vi "Entrenamiento Fuerza 6.vi"(8 "error in (no error)":errorcluster) -> (0 "error out":errorcluster)   [LabVIEW 2014]
panel:
  out "Tiempo Restante":string="15 : 58"
  out "Tiempo Transcurrido":string="04 : 01"
  in  "Reset":bool
  out "Hola":string="4"
  out "Cluster":T1={"Label"="Start", "Cuadriceps"=0, "Isquiotibiales"=0, "Gluteos"=0, "Abdomen"=0, "Lumbares"=0, "Dorsales"=0, "Trapecio"=0, "Pectorales"=35, "Biceps"=87, "Opcional"=0, "Tiempo"=20, "Impulso"=4, "Ruptura"=1, "Frecuencia"=80, "Profundidad"=200, "Ganancia"=0.1, "Master"=54, "Slider"=0}
  out "Master Ind":string="54%"
  in  "Master":bool
  out "Master?":bool
  out "error out 2":errorcluster={"status"=FALSE, "code"=1073676418, "source"="VISA Close in Entrenamiento Fuerza 6.vi"}
  in  "Puerto Serial":refnum<visa-resource-name>="COM25"
  out "Start?":bool
  in  "Start":bool
  in  "Impulso":bool
  in  "Back":bool
  in  "Help":bool
  in  "Slider":i32(slide) scale=0.0..100.0
  out "Horizontal Graduated Bar":i16(slide) scale=0.0..100.0
  in  "Remove Button":bool
  in  "Add Button":bool
  out "Opcional %":string="0%"
  in  "Opcional Bool":bool
  out "Biceps %":string="87%"
  in  "Biceps Bool":bool
  out "Pectorales %":string="35%"
  in  "Pectorales Bool":bool
  out "Trapecio %":string="0%"
  in  "Trapecio Bool":bool
  out "Dorsales %":string="0%"
  in  "Dorsales Bool":bool
  out "Lumbares %":string="0%"
  in  "Lumbares Bool":bool
  out "Abdomen %":string="0%"
  in  "Abdomen Bool":bool
  out "Gluteos %":string="0%"
  in  "Gluteos Bool":bool
  out "Isquiotibiales %":string="0%"
  in  "Isquiotibiales Bool":bool
  out "Cuadríceps %":string="0%"
  in  "Cuadriceps Bool":bool
  out "date/time string":string="26/11/2015 06:09:03 p. m."
  # "Entrenamiento de Fuerza"
  # "Presentación"
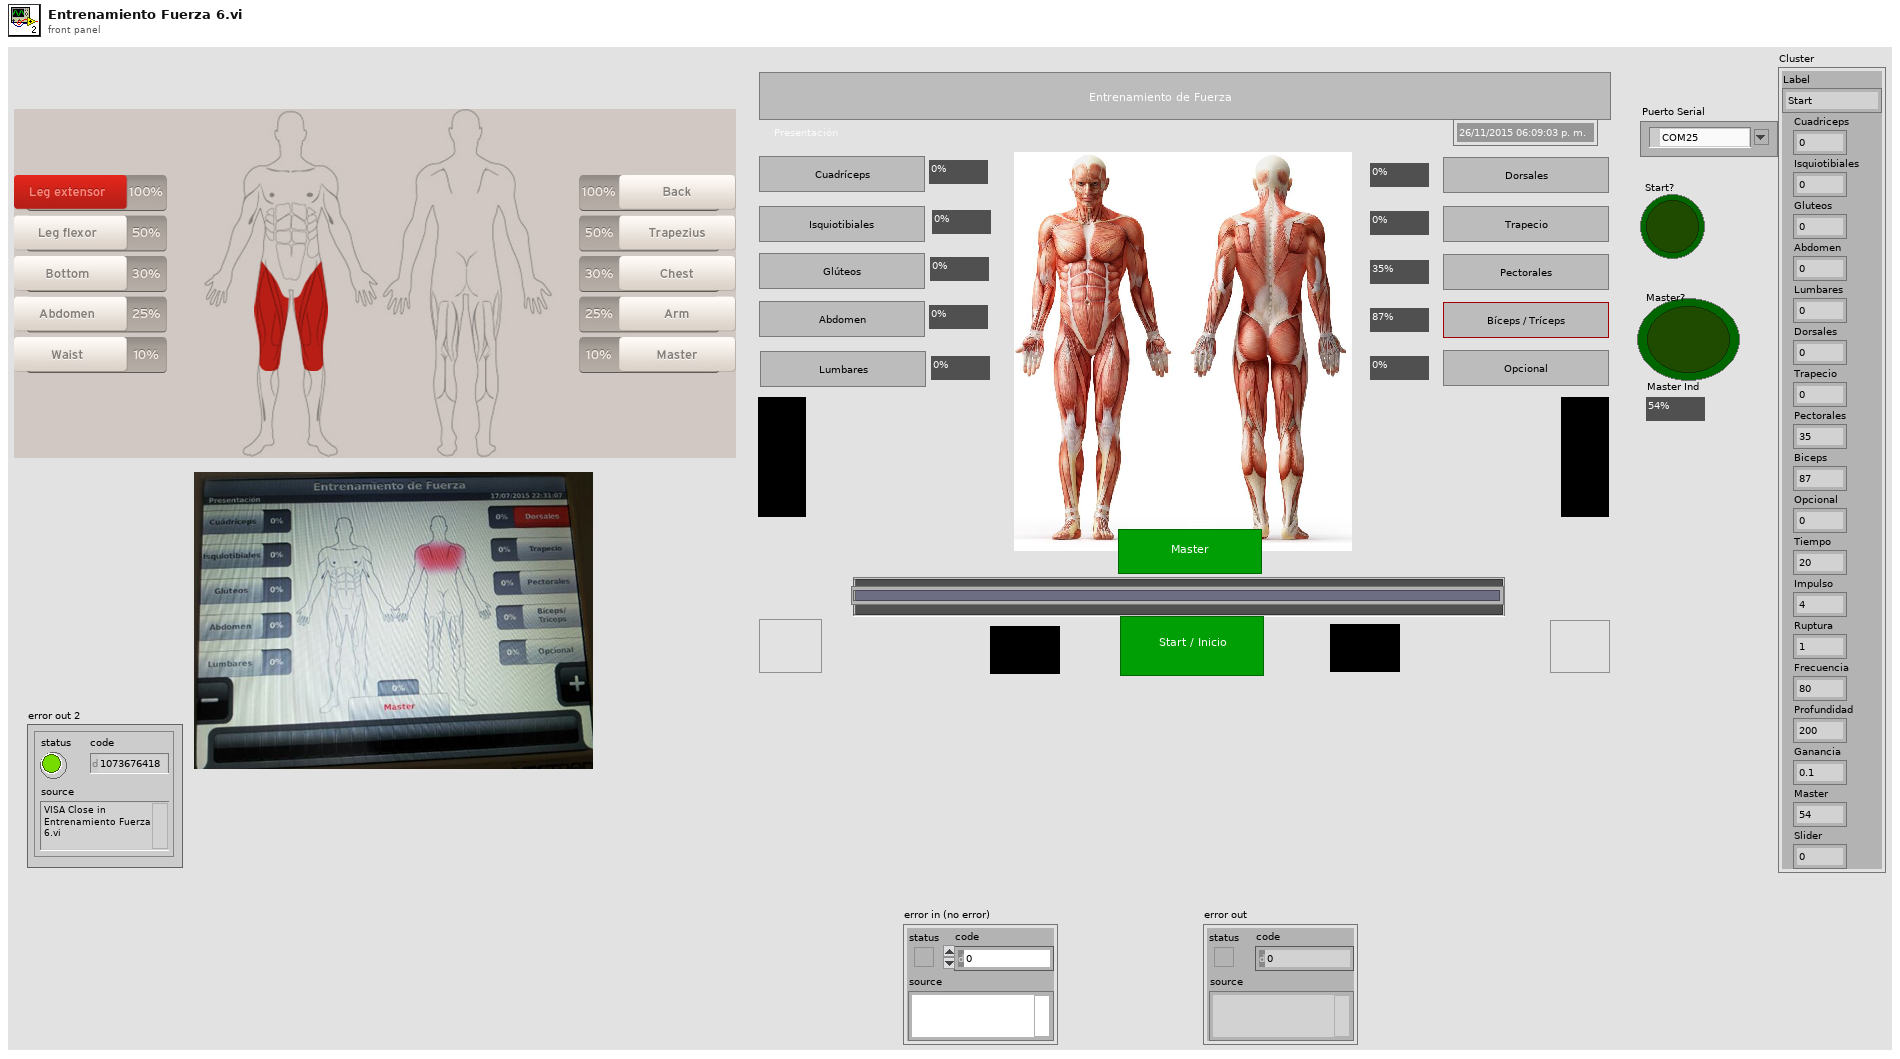
[diagram p1: front panel]
types:
  T1 = cluster{"Label":string, "Cuadriceps":i32, "Isquiotibiales":i32, "Gluteos":i32, "Abdomen":i32, "Lumbares":i32, "Dorsales":i32, "Trapecio":i32, "Pectorales":i32, "Biceps":i32, "Opcional":i32, "Tiempo":i32, "Impulso":i32, "Ruptura":i32, "Frecuencia":i32, "Profundidad":i32, "Ganancia":dbl, "Master":i32, "Slider":i32}
  T2 = cluster{u32, "Boolean Text.Text Colors:Text Color":u32}
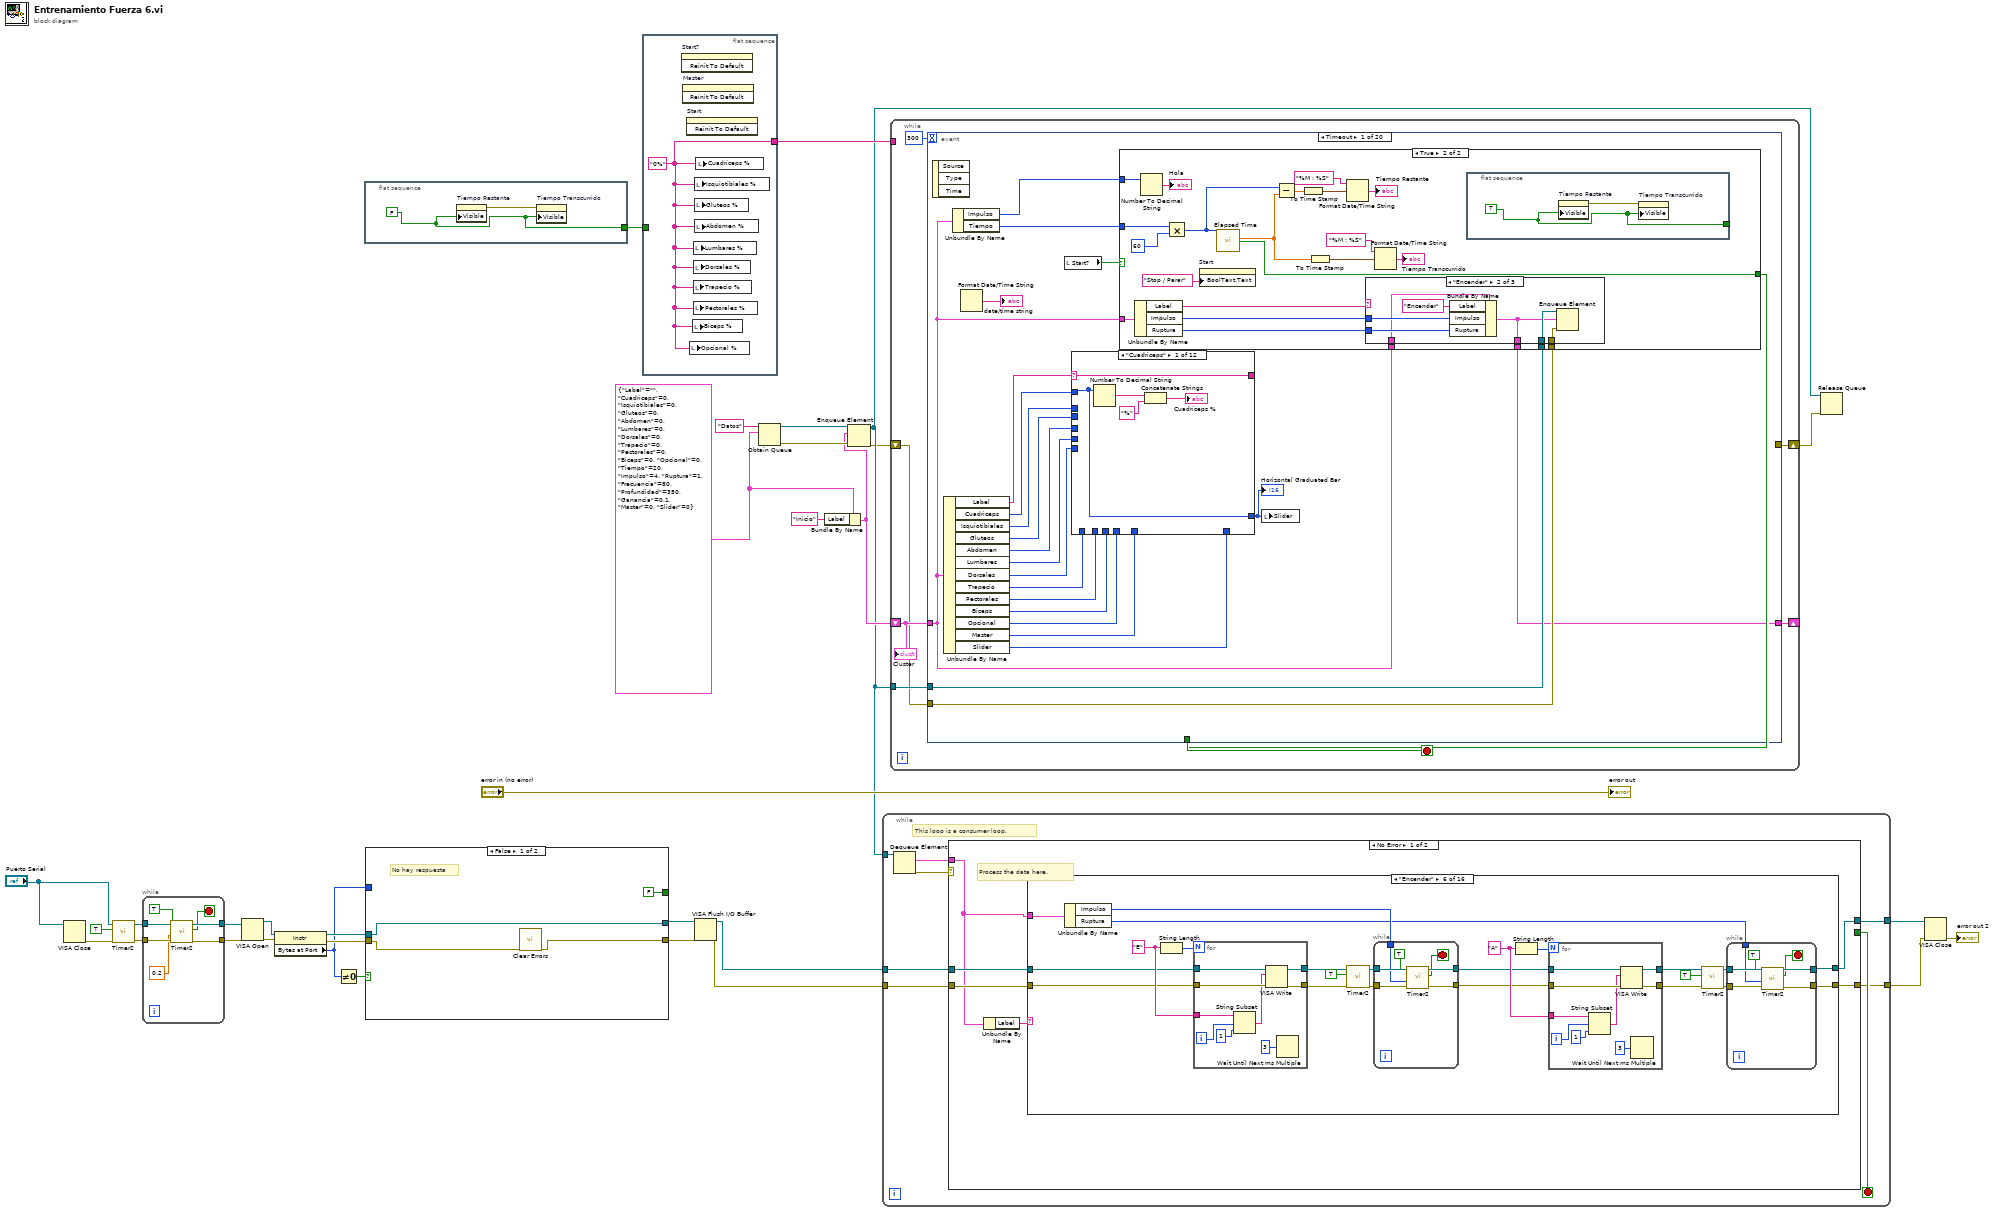
[diagram p0: block diagram]
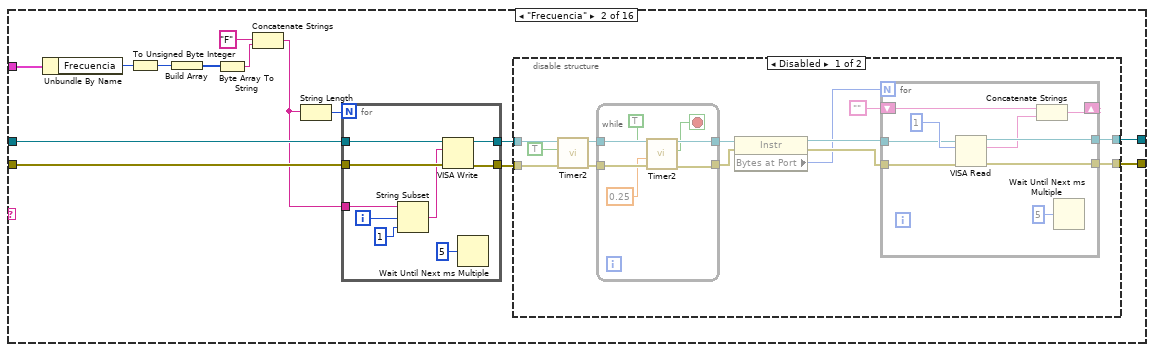
[diagram p3: hidden frame]
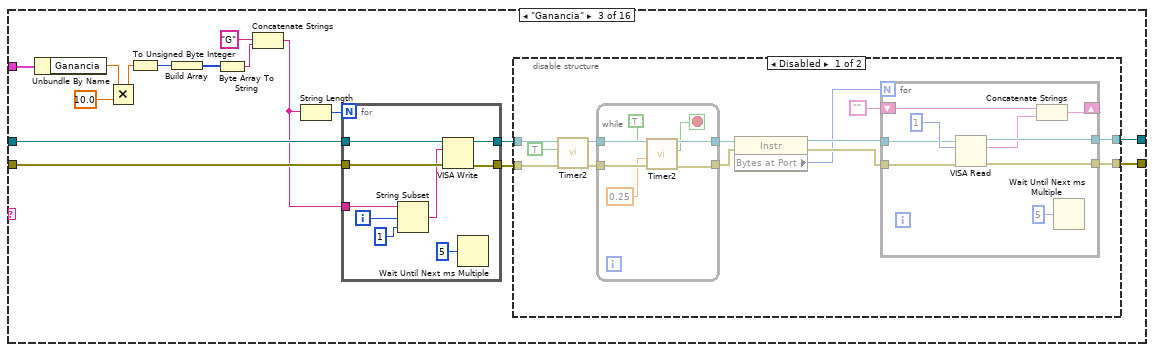
[diagram p5: hidden frame]
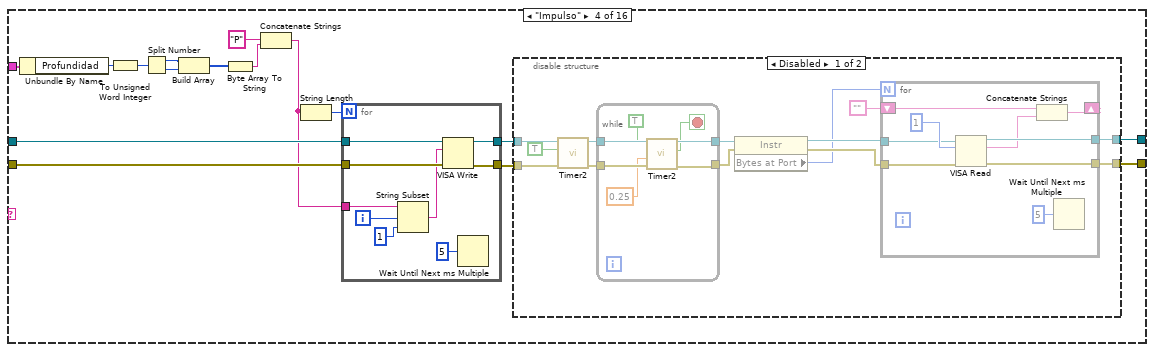
[diagram p7: hidden frame]
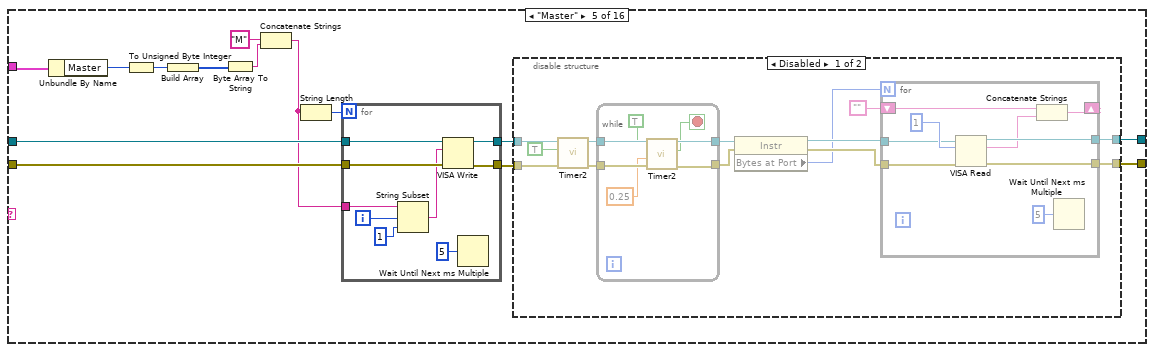
[diagram p9: hidden frame]
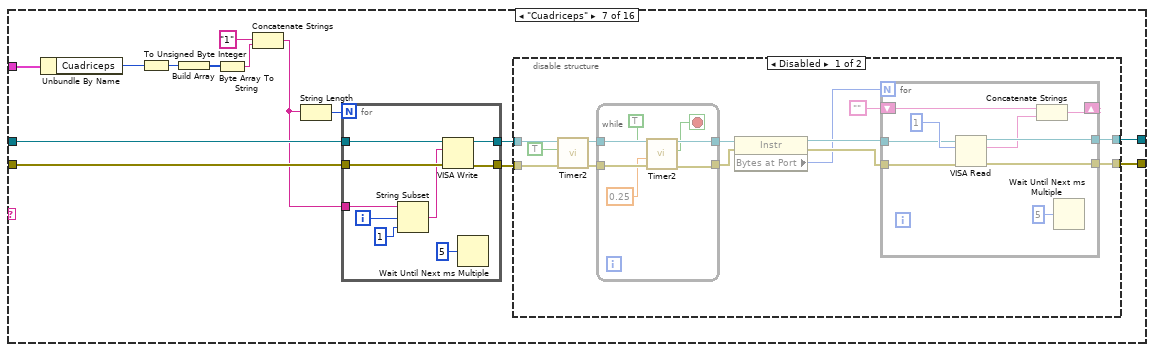
[diagram p11: hidden frame]
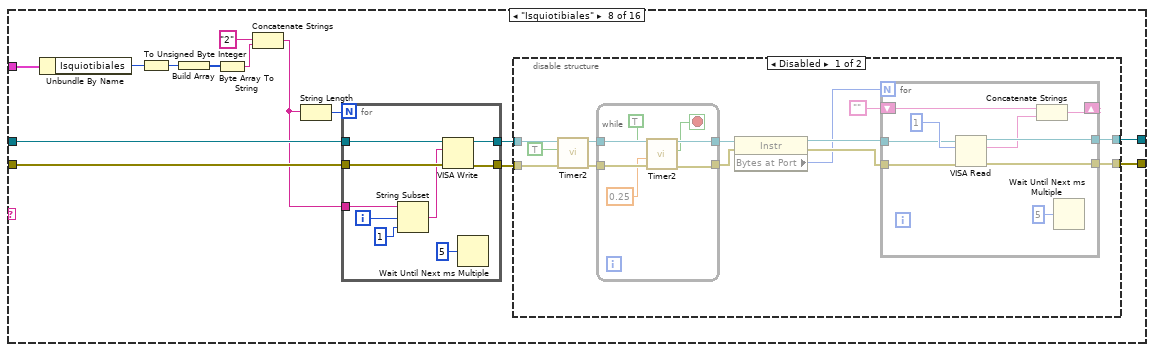
[diagram p13: hidden frame]
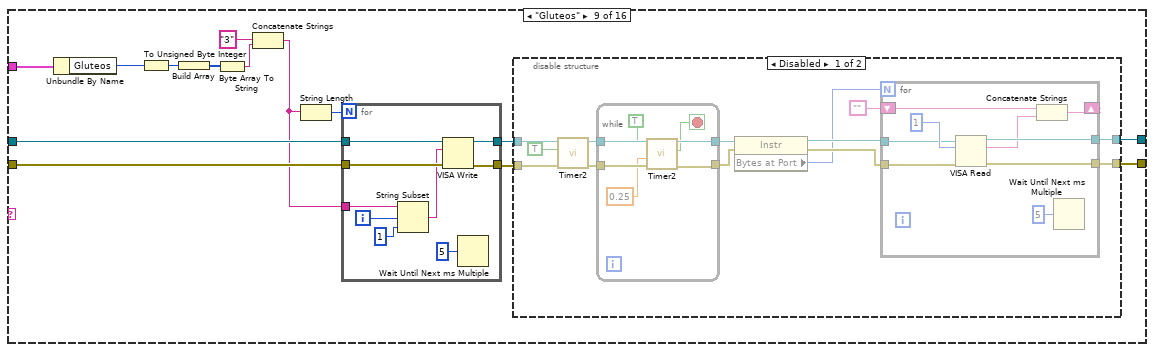
[diagram p15: hidden frame]
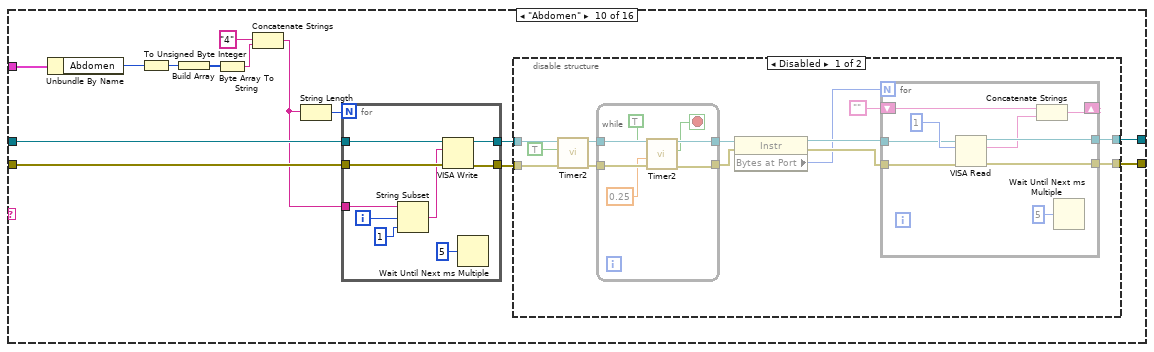
[diagram p17: hidden frame]
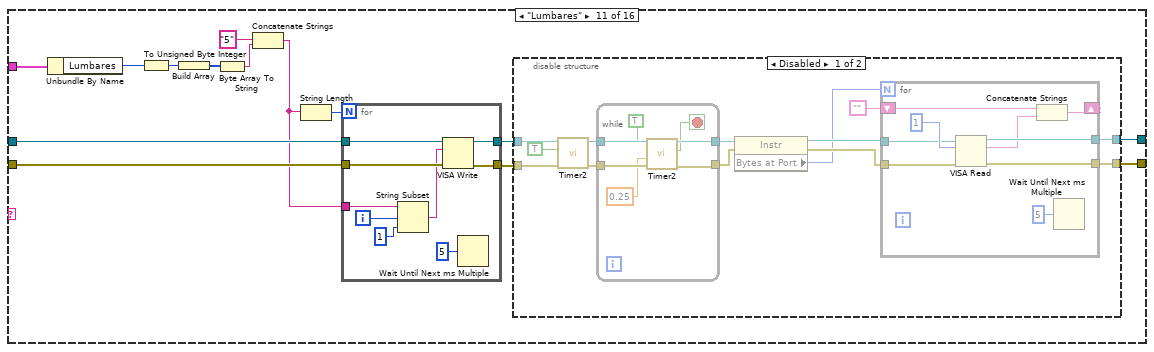
[diagram p19: hidden frame]
diagram:
  w12 = T1 {"Label"="", "Cuadriceps"=0, "Isquiotibiales"=0, "Gluteos"=0, "Abdomen"=0, "Lumbares"=0, "Dorsales"=0, "Trapecio"=0, "Pectorales"=0, "Biceps"=0, "Opcional"=0, "Tiempo"=20, "Impulso"=4, "Ruptura"=1, "Frecuencia"=80, "Profundidad"=350, "Ganancia"=0.1, "Master"=0, "Slider"=0}
  n1 = VISA Close(VISA resource name="Puerto Serial") -> (error out=w27:errorcluster)  [unwired: 1 in]
  n2 = call "Timer2.vi"("error in (no error)"=w27, "Reset"=TRUE) -> ("error out"=w26:errorcluster)  [unwired: 7 in, 2 out]
  n3 = while {
    tunnel: w26 -> [w36]
    tunnel: "Puerto Serial" -> [w37]
    tunnel: [w37] -> w28
    tunnel: [w35] -> w24
    stop <- w34 stop-if-true
    n4 = call "Timer2.vi"("error in (no error)"=w36, "Time Target (s)"=0.2, "Pause"=TRUE) -> ("error out"=w35:errorcluster, "Time has Elapsed"=w34:bool)  [unwired: 6 in, 1 out]
  }
  n5 = VISA Open(error in (no error)=w24, VISA resource name=w28) -> (VISA resource name=w16:refnum<visa-resource-name>, error out=w17:errorcluster)  [unwired: 3 in]
  n6 = property class="Instr"(reference=w16, error in=w17) -> (reference out=w22:refnum<visa-resource-name>, error out=w23:errorcluster, "Bytes at Port"=w20:u32)
  n7 = Not Equal To 0?(x=w20) -> (x != 0?=w21:bool)
  n8 = flat-sequence {
    tunnel: [w38] -> w1
    frame #0 {
      w38 = FALSE ("Visible")
      n9 = property on="Tiempo Restante" class="Str"("Visible"=w38) -> (error out=w39:errorcluster)  [unwired: 2 in, 1 out]
      n10 = property on="Tiempo Transcurrido" class="Str"(error in=w39, "Visible"=w38) -> ()  [unwired: 1 in, 2 out]
    }
  }
  n11 = case shown="False" w21 {
    tunnel: w23 -> [w41 w51]
    tunnel: w22 -> [w43 w50]
    tunnel: w20 -> [_ w49]
    tunnel: [w43 w47] -> w18
    tunnel: [w40 w46] -> w19
    tunnel: [FALSE w45] -> _
    frame False {
      # "No hay respuesta"
      n12 = call <vilib>:"Clear Errors.vi"("error in (no error)"=w41) -> ("error out"=w40:errorcluster)  [unwired: 5 in, 1 out]
    }
    frame True {
      # "Recibe Datos de Respuesta"
      n13 = for {
        N: w49 -> [_]
        tunnel: w51 -> [w60]
        tunnel: w50 -> [w59]
        shift-right: [w54] -> w44
        shift-left: "" -> [w58]
        tunnel: [w57] -> w46
        tunnel: [w56] -> w47
        n14 = VISA Read(VISA resource name=w59, byte count=u32 1, error in (no error)=w60) -> (VISA resource name out=w56:refnum<visa-resource-name>, read buffer=w53:string, error out=w57:errorcluster)  [unwired: 1 out]
        n15 = Concatenate Strings(w58, w53) -> (w54:string)
        n16 = Wait Until Next ms Multiple(millisecond multiple=u32 1) -> ()  [unwired: 1 out]
      }
      n17 = Equal?(x=w44, y="OK") -> (x = y?=w45:bool)
    }
  }
  n18 = flat-sequence {
    tunnel: [w62] -> w15
    tunnel: w1 -> [_]
    frame #0 {
      w62 = "0%" ("Cuadríceps %")
      n19 = invoke on="Start?" class="Bool (strict)" method="Reinit To Default"() -> ()  [unwired: 3 in, 3 out]
      n20 = invoke on="Master" class="Bool (strict)" method="Reinit To Default"() -> ()  [unwired: 3 in, 3 out]
      n21 = invoke on="Start" class="Bool (strict)" method="Reinit To Default"() -> ()  [unwired: 3 in, 3 out]
      n22 = local write "Opcional %"(w62) -> ()
      n23 = local write "Biceps %"(w62) -> ()
      n24 = local write "Trapecio %"(w62) -> ()
      n25 = local write "Pectorales %"(w62) -> ()
      n26 = local write "Lumbares %"(w62) -> ()
      n27 = local write "Dorsales %"(w62) -> ()
      n28 = local write "Isquiotibiales %"(w62) -> ()
      n29 = local write "Gluteos %"(w62) -> ()
      n30 = local write "Abdomen %"(w62) -> ()
      n31 = local write "Cuadríceps %"(w62) -> ()
    }
  }
  n32 = VISA Flush I/O Buffer(VISA resource name=w18, error in (no error)=w19) -> (VISA resource name out=w7:refnum<visa-resource-name>, error out=w6:errorcluster)  [unwired: 1 in]
  n33 = Obtain Queue(name (unnamed)="Datos", element data type=w12) -> (queue out=w13:refnum<queue>, error out=w14:errorcluster)  [unwired: 3 in, 1 out]
  n34 = Bundle By Name(cluster=w12, "Label"="Inicio") -> (w10:T1)
  n35 = Enqueue Element(queue=w13, element=w10, error in (no error)=w14) -> (queue out=w8:refnum<queue>, error out=w3:errorcluster)  [unwired: 1 in, 1 out]
  n36 = while {
    tunnel: w8 -> [w70]
    tunnel: w7 -> [w66]
    tunnel: w6 -> [w65]
    tunnel: [w64] -> w5
    tunnel: [w63] -> w4
    stop <- w67 stop-if-true
    # "This loop is a consumer loop."
    n37 = Dequeue Element(queue=w70) -> (element=w68:T1, error out=w69:errorcluster)  [unwired: 2 in, 2 out]
    n38 = case shown="No Error" w69 {
      tunnel: w68 -> [w71 _]
      tunnel: [_ TRUE] -> w67
      tunnel: w66 -> [w76 w862]
      tunnel: w65 -> [w75 w863]
      tunnel: [w74 w862] -> w64
      tunnel: [w73 w863] -> w63
      frame No Error {
        # "Process the data here."
        n39 = Unbundle By Name(w71) -> ("Label"=w72:string)
        n40 = case shown="\"Encender\"" w72 {
          tunnel: w76 -> [w77 w92 w146 w200 w252 w294 w355 w407 w459 w511 w563 w615 w667 w719 w771 w823]
          tunnel: w75 -> [w78 w91 w145 w199 w251 w293 w354 w406 w458 w510 w562 w614 w666 w718 w770 w822]
          tunnel: [w78 w90 w144 w198 w250 w296 w353 w405 w457 w509 w561 w613 w665 w717 w769 w821] -> w73
          tunnel: [w77 w89 w143 w197 w249 w295 w352 w404 w456 w508 w560 w612 w664 w716 w768 w820] -> w74
          tunnel: w71 -> [_ w81 w136 w190 w239 w311 w344 w396 w448 w500 w552 w604 w656 w708 w760 w812]
          frame "Inicio", Default {
          }
          frame "Frecuencia" {
            n41 = Unbundle By Name(w81) -> ("Frecuencia"=w82:i32)
            n42 = To Unsigned Byte Integer(number=w82) -> (unsigned 8bit integer=w80:u8)
            n43 = Build Array(w80) -> (w79:u8[])
            n44 = Byte Array To String(unsigned byte array=w79) -> (string=w84:string)
            n45 = Concatenate Strings("F", w84) -> (w83:string)
            n46 = String Length(string=w83) -> (length=w88:i32)
            n47 = for {
              N: w88 -> [_]
              tunnel: w91 -> [w130]
              tunnel: w92 -> [w129]
              tunnel: w83 -> [w126]
              tunnel: [w123] -> w86
              tunnel: [w122] -> w87
              i -> [w124]
              n48 = String Subset(string=w126, offset (0)=w124, length (rest)=1 ("length (rest)")) -> (substring=w127:string)
              n49 = VISA Write(VISA resource name=w129, write buffer=w127, error in (no error)=w130) -> (VISA resource name out=w122:refnum<visa-resource-name>, error out=w123:errorcluster)  [unwired: 1 out]
              n50 = Wait Until Next ms Multiple(millisecond multiple=u32 5) -> ()  [unwired: 1 out]
            }
            n51 = disable-structure shown="Disabled" {
              disable-tunnel: [w104 w120] -> w90
              disable-tunnel: [w103 w121] -> w89
              disable-tunnel: w87 -> [w98 w121]
              disable-tunnel: w86 -> [w94 w120]
              frame Disabled {
                n52 = call "Timer2.vi"("error in (no error)"=w94, "Reset"=TRUE) -> ("error out"=w93:errorcluster)  [unwired: 7 in, 2 out]
                n53 = while {
                  tunnel: w98 -> [w110]
                  tunnel: [w110] -> w97
                  tunnel: [w108] -> w96
                  tunnel: w93 -> [w109]
                  stop <- w107 stop-if-true
                  n54 = call "Timer2.vi"("error in (no error)"=w109, "Time Target (s)"=0.25, "Pause"=TRUE) -> ("error out"=w108:errorcluster, "Time has Elapsed"=w107:bool)  [unwired: 6 in, 1 out]
                }
                n55 = property class="Instr"(reference=w97, error in=w96) -> (reference out=w101:refnum<visa-resource-name>, error out=w100:errorcluster, "Bytes at Port"=w99:u32)
                n56 = for {
                  N: w99 -> [_]
                  tunnel: w100 -> [w118]
                  tunnel: w101 -> [w117]
                  shift-right: [w112] -> _
                  shift-left: "" -> [w116]
                  tunnel: [w115] -> w104
                  tunnel: [w114] -> w103
                  n57 = VISA Read(VISA resource name=w117, byte count=u32 1, error in (no error)=w118) -> (VISA resource name out=w114:refnum<visa-resource-name>, read buffer=w111:string, error out=w115:errorcluster)  [unwired: 1 out]
                  n58 = Concatenate Strings(w116, w111) -> (w112:string)
                  n59 = Wait Until Next ms Multiple(millisecond multiple=u32 5) -> ()  [unwired: 1 out]
                }
              }
              frame Enabled {
              }
            }
          }
          frame "Ganancia" {
            n60 = Unbundle By Name(w136) -> ("Ganancia"=w132:dbl)
            n61 = Multiply(x=w132, y=10.0) -> (x*y=w133:dbl)
            n62 = To Unsigned Byte Integer(number=w133) -> (unsigned 8bit integer=w135:u8)
            n63 = Build Array(w135) -> (w134:u8[])
            n64 = Byte Array To String(unsigned byte array=w134) -> (string=w138:string)
            n65 = Concatenate Strings("G", w138) -> (w137:string)
            n66 = String Length(string=w137) -> (length=w142:i32)
            n67 = for {
              N: w142 -> [_]
              tunnel: w145 -> [w184]
              tunnel: w146 -> [w183]
              tunnel: w137 -> [w180]
              tunnel: [w177] -> w140
              tunnel: [w176] -> w141
              i -> [w178]
              n68 = String Subset(string=w180, offset (0)=w178, length (rest)=1 ("length (rest)")) -> (substring=w181:string)
              n69 = VISA Write(VISA resource name=w183, write buffer=w181, error in (no error)=w184) -> (VISA resource name out=w176:refnum<visa-resource-name>, error out=w177:errorcluster)  [unwired: 1 out]
              n70 = Wait Until Next ms Multiple(millisecond multiple=u32 5) -> ()  [unwired: 1 out]
            }
            n71 = disable-structure shown="Disabled" {
              disable-tunnel: [w158 w174] -> w144
              disable-tunnel: [w157 w175] -> w143
              disable-tunnel: w141 -> [w152 w175]
              disable-tunnel: w140 -> [w148 w174]
              frame Disabled {
                n72 = call "Timer2.vi"("error in (no error)"=w148, "Reset"=TRUE) -> ("error out"=w147:errorcluster)  [unwired: 7 in, 2 out]
                n73 = while {
                  tunnel: w152 -> [w164]
                  tunnel: [w164] -> w151
                  tunnel: [w162] -> w150
                  tunnel: w147 -> [w163]
                  stop <- w161 stop-if-true
                  n74 = call "Timer2.vi"("error in (no error)"=w163, "Time Target (s)"=0.25, "Pause"=TRUE) -> ("error out"=w162:errorcluster, "Time has Elapsed"=w161:bool)  [unwired: 6 in, 1 out]
                }
                n75 = property class="Instr"(reference=w151, error in=w150) -> (reference out=w155:refnum<visa-resource-name>, error out=w154:errorcluster, "Bytes at Port"=w153:u32)
                n76 = for {
                  N: w153 -> [_]
                  tunnel: w154 -> [w172]
                  tunnel: w155 -> [w171]
                  shift-right: [w166] -> _
                  shift-left: "" -> [w170]
                  tunnel: [w169] -> w158
                  tunnel: [w168] -> w157
                  n77 = VISA Read(VISA resource name=w171, byte count=u32 1, error in (no error)=w172) -> (VISA resource name out=w168:refnum<visa-resource-name>, read buffer=w165:string, error out=w169:errorcluster)  [unwired: 1 out]
                  n78 = Concatenate Strings(w170, w165) -> (w166:string)
                  n79 = Wait Until Next ms Multiple(millisecond multiple=u32 5) -> ()  [unwired: 1 out]
                }
              }
              frame Enabled {
              }
            }
          }
          frame "Impulso" {
            n80 = Unbundle By Name(w190) -> ("Profundidad"=w187:i32)
            n81 = To Unsigned Word Integer(number=w187) -> (unsigned 16bit integer=w186:u16)
            n82 = Split Number(x=w186) -> (hi(x)=w189:u8, lo(x)=w188:u8)
            n83 = Build Array(w189, w188) -> (w185:u8[])
            n84 = Byte Array To String(unsigned byte array=w185) -> (string=w192:string)
            n85 = Concatenate Strings("P", w192) -> (w191:string)
            n86 = String Length(string=w191) -> (length=w196:i32)
            n87 = for {
              N: w196 -> [_]
              tunnel: w199 -> [w238]
              tunnel: w200 -> [w237]
              tunnel: w191 -> [w234]
              tunnel: [w231] -> w194
              tunnel: [w230] -> w195
              i -> [w232]
              n88 = String Subset(string=w234, offset (0)=w232, length (rest)=1 ("length (rest)")) -> (substring=w235:string)
              n89 = VISA Write(VISA resource name=w237, write buffer=w235, error in (no error)=w238) -> (VISA resource name out=w230:refnum<visa-resource-name>, error out=w231:errorcluster)  [unwired: 1 out]
              n90 = Wait Until Next ms Multiple(millisecond multiple=u32 5) -> ()  [unwired: 1 out]
            }
            n91 = disable-structure shown="Disabled" {
              disable-tunnel: [w212 w228] -> w198
              disable-tunnel: [w211 w229] -> w197
              disable-tunnel: w195 -> [w206 w229]
              disable-tunnel: w194 -> [w202 w228]
              frame Disabled {
                n92 = call "Timer2.vi"("error in (no error)"=w202, "Reset"=TRUE) -> ("error out"=w201:errorcluster)  [unwired: 7 in, 2 out]
                n93 = while {
                  tunnel: w206 -> [w218]
                  tunnel: [w218] -> w205
                  tunnel: [w216] -> w204
                  tunnel: w201 -> [w217]
                  stop <- w215 stop-if-true
                  n94 = call "Timer2.vi"("error in (no error)"=w217, "Time Target (s)"=0.25, "Pause"=TRUE) -> ("error out"=w216:errorcluster, "Time has Elapsed"=w215:bool)  [unwired: 6 in, 1 out]
                }
                n95 = property class="Instr"(reference=w205, error in=w204) -> (reference out=w209:refnum<visa-resource-name>, error out=w208:errorcluster, "Bytes at Port"=w207:u32)
                n96 = for {
                  N: w207 -> [_]
                  tunnel: w208 -> [w226]
                  tunnel: w209 -> [w225]
                  shift-right: [w220] -> _
                  shift-left: "" -> [w224]
                  tunnel: [w223] -> w212
                  tunnel: [w222] -> w211
                  n97 = VISA Read(VISA resource name=w225, byte count=u32 1, error in (no error)=w226) -> (VISA resource name out=w222:refnum<visa-resource-name>, read buffer=w219:string, error out=w223:errorcluster)  [unwired: 1 out]
                  n98 = Concatenate Strings(w224, w219) -> (w220:string)
                  n99 = Wait Until Next ms Multiple(millisecond multiple=u32 5) -> ()  [unwired: 1 out]
                }
              }
              frame Enabled {
              }
            }
          }
          frame "Master" {
            n100 = Unbundle By Name(w239) -> ("Master"=w242:i32)
            n101 = To Unsigned Byte Integer(number=w242) -> (unsigned 8bit integer=w241:u8)
            n102 = Build Array(w241) -> (w240:u8[])
            n103 = Byte Array To String(unsigned byte array=w240) -> (string=w244:string)
            n104 = Concatenate Strings("M", w244) -> (w243:string)
            n105 = String Length(string=w243) -> (length=w248:i32)
            n106 = for {
              N: w248 -> [_]
              tunnel: w251 -> [w290]
              tunnel: w252 -> [w289]
              tunnel: w243 -> [w286]
              tunnel: [w283] -> w246
              tunnel: [w282] -> w247
              i -> [w284]
              n107 = String Subset(string=w286, offset (0)=w284, length (rest)=1 ("length (rest)")) -> (substring=w287:string)
              n108 = VISA Write(VISA resource name=w289, write buffer=w287, error in (no error)=w290) -> (VISA resource name out=w282:refnum<visa-resource-name>, error out=w283:errorcluster)  [unwired: 1 out]
              n109 = Wait Until Next ms Multiple(millisecond multiple=u32 5) -> ()  [unwired: 1 out]
            }
            n110 = disable-structure shown="Disabled" {
              disable-tunnel: [w264 w280] -> w250
              disable-tunnel: [w263 w281] -> w249
              disable-tunnel: w247 -> [w258 w281]
              disable-tunnel: w246 -> [w254 w280]
              frame Disabled {
                n111 = call "Timer2.vi"("error in (no error)"=w254, "Reset"=TRUE) -> ("error out"=w253:errorcluster)  [unwired: 7 in, 2 out]
                n112 = while {
                  tunnel: w258 -> [w270]
                  tunnel: [w270] -> w257
                  tunnel: [w268] -> w256
                  tunnel: w253 -> [w269]
                  stop <- w267 stop-if-true
                  n113 = call "Timer2.vi"("error in (no error)"=w269, "Time Target (s)"=0.25, "Pause"=TRUE) -> ("error out"=w268:errorcluster, "Time has Elapsed"=w267:bool)  [unwired: 6 in, 1 out]
                }
                n114 = property class="Instr"(reference=w257, error in=w256) -> (reference out=w261:refnum<visa-resource-name>, error out=w260:errorcluster, "Bytes at Port"=w259:u32)
                n115 = for {
                  N: w259 -> [_]
                  tunnel: w260 -> [w278]
                  tunnel: w261 -> [w277]
                  shift-right: [w272] -> _
                  shift-left: "" -> [w276]
                  tunnel: [w275] -> w264
                  tunnel: [w274] -> w263
                  n116 = VISA Read(VISA resource name=w277, byte count=u32 1, error in (no error)=w278) -> (VISA resource name out=w274:refnum<visa-resource-name>, read buffer=w271:string, error out=w275:errorcluster)  [unwired: 1 out]
                  n117 = Concatenate Strings(w276, w271) -> (w272:string)
                  n118 = Wait Until Next ms Multiple(millisecond multiple=u32 5) -> ()  [unwired: 1 out]
                }
              }
              frame Enabled {
              }
            }
          }
          frame "Encender" {
            w301 = "A"
            w307 = "E"
            n119 = Unbundle By Name(w311) -> ("Impulso"=w292:i32, "Ruptura"=w291:i32)
            n120 = String Length(string=w307) -> (length=w310:i32)
            n121 = for {
              N: w310 -> [_]
              tunnel: w293 -> [w341]
              tunnel: w294 -> [w340]
              tunnel: w307 -> [w337]
              tunnel: [w334] -> w308
              tunnel: [w333] -> w309
              i -> [w335]
              n122 = String Subset(string=w337, offset (0)=w335, length (rest)=1 ("length (rest)")) -> (substring=w338:string)
              n123 = VISA Write(VISA resource name=w340, write buffer=w338, error in (no error)=w341) -> (VISA resource name out=w333:refnum<visa-resource-name>, error out=w334:errorcluster)  [unwired: 1 out]
              n124 = Wait Until Next ms Multiple(millisecond multiple=u32 3) -> ()  [unwired: 1 out]
            }
            n125 = call "Timer2.vi"("error in (no error)"=w308, "Reset"=TRUE) -> ("error out"=w305:errorcluster)  [unwired: 7 in, 2 out]
            n126 = while {
              tunnel: w309 -> [w332]
              tunnel: [w332] -> w298
              tunnel: [w330] -> w297
              tunnel: w305 -> [w331]
              tunnel: w292 -> [w327]
              stop <- w329 stop-if-true
              n127 = call "Timer2.vi"("error in (no error)"=w331, "Time Target (s)"=w327, "Pause"=TRUE) -> ("error out"=w330:errorcluster, "Time has Elapsed"=w329:bool)  [unwired: 6 in, 1 out]
            }
            n128 = String Length(string=w301) -> (length=w304:i32)
            n129 = for {
              N: w304 -> [_]
              tunnel: w297 -> [w326]
              tunnel: w298 -> [w325]
              tunnel: w301 -> [w322]
              tunnel: [w319] -> w302
              tunnel: [w318] -> w303
              i -> [w320]
              n130 = String Subset(string=w322, offset (0)=w320, length (rest)=1 ("length (rest)")) -> (substring=w323:string)
              n131 = VISA Write(VISA resource name=w325, write buffer=w323, error in (no error)=w326) -> (VISA resource name out=w318:refnum<visa-resource-name>, error out=w319:errorcluster)  [unwired: 1 out]
              n132 = Wait Until Next ms Multiple(millisecond multiple=u32 3) -> ()  [unwired: 1 out]
            }
            n133 = call "Timer2.vi"("error in (no error)"=w302, "Reset"=TRUE) -> ("error out"=w299:errorcluster)  [unwired: 7 in, 2 out]
            n134 = while {
              tunnel: w303 -> [w317]
              tunnel: [w317] -> w295
              tunnel: [w315] -> w296
              tunnel: w299 -> [w316]
              tunnel: w291 -> [w312]
              stop <- w314 stop-if-true
              n135 = call "Timer2.vi"("error in (no error)"=w316, "Time Target (s)"=w312, "Pause"=TRUE) -> ("error out"=w315:errorcluster, "Time has Elapsed"=w314:bool)  [unwired: 6 in, 1 out]
            }
          }
          frame "Cuadriceps" {
            n136 = Unbundle By Name(w344) -> ("Cuadriceps"=w342:i32)
            n137 = To Unsigned Byte Integer(number=w342) -> (unsigned 8bit integer=w343:u8)
            n138 = Build Array(w343) -> (w348:u8[])
            n139 = Byte Array To String(unsigned byte array=w348) -> (string=w346:string)
            n140 = Concatenate Strings("1", w346) -> (w345:string)
            n141 = String Length(string=w345) -> (length=w351:i32)
            n142 = for {
              N: w351 -> [_]
              tunnel: w354 -> [w393]
              tunnel: w355 -> [w392]
              tunnel: w345 -> [w389]
              tunnel: [w386] -> w349
              tunnel: [w385] -> w350
              i -> [w387]
              n143 = String Subset(string=w389, offset (0)=w387, length (rest)=1 ("length (rest)")) -> (substring=w390:string)
              n144 = VISA Write(VISA resource name=w392, write buffer=w390, error in (no error)=w393) -> (VISA resource name out=w385:refnum<visa-resource-name>, error out=w386:errorcluster)  [unwired: 1 out]
              n145 = Wait Until Next ms Multiple(millisecond multiple=u32 5) -> ()  [unwired: 1 out]
            }
            n146 = disable-structure shown="Disabled" {
              disable-tunnel: [w367 w383] -> w353
              disable-tunnel: [w366 w384] -> w352
              disable-tunnel: w350 -> [w361 w384]
              disable-tunnel: w349 -> [w357 w383]
              frame Disabled {
                n147 = call "Timer2.vi"("error in (no error)"=w357, "Reset"=TRUE) -> ("error out"=w356:errorcluster)  [unwired: 7 in, 2 out]
                n148 = while {
                  tunnel: w361 -> [w373]
                  tunnel: [w373] -> w360
                  tunnel: [w371] -> w359
                  tunnel: w356 -> [w372]
                  stop <- w370 stop-if-true
                  n149 = call "Timer2.vi"("error in (no error)"=w372, "Time Target (s)"=0.25, "Pause"=TRUE) -> ("error out"=w371:errorcluster, "Time has Elapsed"=w370:bool)  [unwired: 6 in, 1 out]
                }
                n150 = property class="Instr"(reference=w360, error in=w359) -> (reference out=w364:refnum<visa-resource-name>, error out=w363:errorcluster, "Bytes at Port"=w362:u32)
                n151 = for {
                  N: w362 -> [_]
                  tunnel: w363 -> [w381]
                  tunnel: w364 -> [w380]
                  shift-right: [w375] -> _
                  shift-left: "" -> [w379]
                  tunnel: [w378] -> w367
                  tunnel: [w377] -> w366
                  n152 = VISA Read(VISA resource name=w380, byte count=u32 1, error in (no error)=w381) -> (VISA resource name out=w377:refnum<visa-resource-name>, read buffer=w374:string, error out=w378:errorcluster)  [unwired: 1 out]
                  n153 = Concatenate Strings(w379, w374) -> (w375:string)
                  n154 = Wait Until Next ms Multiple(millisecond multiple=u32 5) -> ()  [unwired: 1 out]
                }
              }
              frame Enabled {
              }
            }
          }
          frame "Isquiotibiales" {
            n155 = Unbundle By Name(w396) -> ("Isquiotibiales"=w394:i32)
            n156 = To Unsigned Byte Integer(number=w394) -> (unsigned 8bit integer=w395:u8)
            n157 = Build Array(w395) -> (w400:u8[])
            n158 = Byte Array To String(unsigned byte array=w400) -> (string=w398:string)
            n159 = Concatenate Strings("2", w398) -> (w397:string)
            n160 = String Length(string=w397) -> (length=w403:i32)
            n161 = for {
              N: w403 -> [_]
              tunnel: w406 -> [w445]
              tunnel: w407 -> [w444]
              tunnel: w397 -> [w441]
              tunnel: [w438] -> w401
              tunnel: [w437] -> w402
              i -> [w439]
              n162 = String Subset(string=w441, offset (0)=w439, length (rest)=1 ("length (rest)")) -> (substring=w442:string)
              n163 = VISA Write(VISA resource name=w444, write buffer=w442, error in (no error)=w445) -> (VISA resource name out=w437:refnum<visa-resource-name>, error out=w438:errorcluster)  [unwired: 1 out]
              n164 = Wait Until Next ms Multiple(millisecond multiple=u32 5) -> ()  [unwired: 1 out]
            }
            n165 = disable-structure shown="Disabled" {
              disable-tunnel: [w419 w435] -> w405
              disable-tunnel: [w418 w436] -> w404
              disable-tunnel: w402 -> [w413 w436]
              disable-tunnel: w401 -> [w409 w435]
              frame Disabled {
                n166 = call "Timer2.vi"("error in (no error)"=w409, "Reset"=TRUE) -> ("error out"=w408:errorcluster)  [unwired: 7 in, 2 out]
                n167 = while {
                  tunnel: w413 -> [w425]
                  tunnel: [w425] -> w412
                  tunnel: [w423] -> w411
                  tunnel: w408 -> [w424]
                  stop <- w422 stop-if-true
                  n168 = call "Timer2.vi"("error in (no error)"=w424, "Time Target (s)"=0.25, "Pause"=TRUE) -> ("error out"=w423:errorcluster, "Time has Elapsed"=w422:bool)  [unwired: 6 in, 1 out]
                }
                n169 = property class="Instr"(reference=w412, error in=w411) -> (reference out=w416:refnum<visa-resource-name>, error out=w415:errorcluster, "Bytes at Port"=w414:u32)
                n170 = for {
                  N: w414 -> [_]
                  tunnel: w415 -> [w433]
                  tunnel: w416 -> [w432]
                  shift-right: [w427] -> _
                  shift-left: "" -> [w431]
                  tunnel: [w430] -> w419
                  tunnel: [w429] -> w418
                  n171 = VISA Read(VISA resource name=w432, byte count=u32 1, error in (no error)=w433) -> (VISA resource name out=w429:refnum<visa-resource-name>, read buffer=w426:string, error out=w430:errorcluster)  [unwired: 1 out]
                  n172 = Concatenate Strings(w431, w426) -> (w427:string)
                  n173 = Wait Until Next ms Multiple(millisecond multiple=u32 5) -> ()  [unwired: 1 out]
                }
              }
              frame Enabled {
              }
            }
          }
          frame "Gluteos" {
            n174 = Unbundle By Name(w448) -> ("Gluteos"=w446:i32)
            n175 = To Unsigned Byte Integer(number=w446) -> (unsigned 8bit integer=w447:u8)
            n176 = Build Array(w447) -> (w452:u8[])
            n177 = Byte Array To String(unsigned byte array=w452) -> (string=w450:string)
            n178 = Concatenate Strings("3", w450) -> (w449:string)
            n179 = String Length(string=w449) -> (length=w455:i32)
            n180 = for {
              N: w455 -> [_]
              tunnel: w458 -> [w497]
              tunnel: w459 -> [w496]
              tunnel: w449 -> [w493]
              tunnel: [w490] -> w453
              tunnel: [w489] -> w454
              i -> [w491]
              n181 = String Subset(string=w493, offset (0)=w491, length (rest)=1 ("length (rest)")) -> (substring=w494:string)
              n182 = VISA Write(VISA resource name=w496, write buffer=w494, error in (no error)=w497) -> (VISA resource name out=w489:refnum<visa-resource-name>, error out=w490:errorcluster)  [unwired: 1 out]
              n183 = Wait Until Next ms Multiple(millisecond multiple=u32 5) -> ()  [unwired: 1 out]
            }
            n184 = disable-structure shown="Disabled" {
              disable-tunnel: [w471 w487] -> w457
              disable-tunnel: [w470 w488] -> w456
              disable-tunnel: w454 -> [w465 w488]
              disable-tunnel: w453 -> [w461 w487]
              frame Disabled {
                n185 = call "Timer2.vi"("error in (no error)"=w461, "Reset"=TRUE) -> ("error out"=w460:errorcluster)  [unwired: 7 in, 2 out]
                n186 = while {
                  tunnel: w465 -> [w477]
                  tunnel: [w477] -> w464
                  tunnel: [w475] -> w463
                  tunnel: w460 -> [w476]
                  stop <- w474 stop-if-true
                  n187 = call "Timer2.vi"("error in (no error)"=w476, "Time Target (s)"=0.25, "Pause"=TRUE) -> ("error out"=w475:errorcluster, "Time has Elapsed"=w474:bool)  [unwired: 6 in, 1 out]
                }
                n188 = property class="Instr"(reference=w464, error in=w463) -> (reference out=w468:refnum<visa-resource-name>, error out=w467:errorcluster, "Bytes at Port"=w466:u32)
                n189 = for {
                  N: w466 -> [_]
                  tunnel: w467 -> [w485]
                  tunnel: w468 -> [w484]
                  shift-right: [w479] -> _
                  shift-left: "" -> [w483]
                  tunnel: [w482] -> w471
                  tunnel: [w481] -> w470
                  n190 = VISA Read(VISA resource name=w484, byte count=u32 1, error in (no error)=w485) -> (VISA resource name out=w481:refnum<visa-resource-name>, read buffer=w478:string, error out=w482:errorcluster)  [unwired: 1 out]
                  n191 = Concatenate Strings(w483, w478) -> (w479:string)
                  n192 = Wait Until Next ms Multiple(millisecond multiple=u32 5) -> ()  [unwired: 1 out]
                }
              }
              frame Enabled {
              }
            }
          }
          frame "Abdomen" {
            n193 = Unbundle By Name(w500) -> ("Abdomen"=w498:i32)
            n194 = To Unsigned Byte Integer(number=w498) -> (unsigned 8bit integer=w499:u8)
            n195 = Build Array(w499) -> (w504:u8[])
            n196 = Byte Array To String(unsigned byte array=w504) -> (string=w502:string)
            n197 = Concatenate Strings("4", w502) -> (w501:string)
            n198 = String Length(string=w501) -> (length=w507:i32)
            n199 = for {
              N: w507 -> [_]
              tunnel: w510 -> [w549]
              tunnel: w511 -> [w548]
              tunnel: w501 -> [w545]
              tunnel: [w542] -> w505
              tunnel: [w541] -> w506
              i -> [w543]
              n200 = String Subset(string=w545, offset (0)=w543, length (rest)=1 ("length (rest)")) -> (substring=w546:string)
              n201 = VISA Write(VISA resource name=w548, write buffer=w546, error in (no error)=w549) -> (VISA resource name out=w541:refnum<visa-resource-name>, error out=w542:errorcluster)  [unwired: 1 out]
              n202 = Wait Until Next ms Multiple(millisecond multiple=u32 5) -> ()  [unwired: 1 out]
            }
            n203 = disable-structure shown="Disabled" {
              disable-tunnel: [w523 w539] -> w509
              disable-tunnel: [w522 w540] -> w508
              disable-tunnel: w506 -> [w517 w540]
              disable-tunnel: w505 -> [w513 w539]
              frame Disabled {
                n204 = call "Timer2.vi"("error in (no error)"=w513, "Reset"=TRUE) -> ("error out"=w512:errorcluster)  [unwired: 7 in, 2 out]
                n205 = while {
                  tunnel: w517 -> [w529]
                  tunnel: [w529] -> w516
                  tunnel: [w527] -> w515
                  tunnel: w512 -> [w528]
                  stop <- w526 stop-if-true
                  n206 = call "Timer2.vi"("error in (no error)"=w528, "Time Target (s)"=0.25, "Pause"=TRUE) -> ("error out"=w527:errorcluster, "Time has Elapsed"=w526:bool)  [unwired: 6 in, 1 out]
                }
                n207 = property class="Instr"(reference=w516, error in=w515) -> (reference out=w520:refnum<visa-resource-name>, error out=w519:errorcluster, "Bytes at Port"=w518:u32)
                n208 = for {
                  N: w518 -> [_]
                  tunnel: w519 -> [w537]
                  tunnel: w520 -> [w536]
                  shift-right: [w531] -> _
                  shift-left: "" -> [w535]
                  tunnel: [w534] -> w523
                  tunnel: [w533] -> w522
                  n209 = VISA Read(VISA resource name=w536, byte count=u32 1, error in (no error)=w537) -> (VISA resource name out=w533:refnum<visa-resource-name>, read buffer=w530:string, error out=w534:errorcluster)  [unwired: 1 out]
                  n210 = Concatenate Strings(w535, w530) -> (w531:string)
                  n211 = Wait Until Next ms Multiple(millisecond multiple=u32 5) -> ()  [unwired: 1 out]
                }
              }
              frame Enabled {
              }
            }
          }
          frame "Lumbares" {
            n212 = Unbundle By Name(w552) -> ("Lumbares"=w550:i32)
            n213 = To Unsigned Byte Integer(number=w550) -> (unsigned 8bit integer=w551:u8)
            n214 = Build Array(w551) -> (w556:u8[])
            n215 = Byte Array To String(unsigned byte array=w556) -> (string=w554:string)
            n216 = Concatenate Strings("5", w554) -> (w553:string)
            n217 = String Length(string=w553) -> (length=w559:i32)
            n218 = for {
              N: w559 -> [_]
              tunnel: w562 -> [w601]
              tunnel: w563 -> [w600]
              tunnel: w553 -> [w597]
              tunnel: [w594] -> w557
              tunnel: [w593] -> w558
              i -> [w595]
              n219 = String Subset(string=w597, offset (0)=w595, length (rest)=1 ("length (rest)")) -> (substring=w598:string)
              n220 = VISA Write(VISA resource name=w600, write buffer=w598, error in (no error)=w601) -> (VISA resource name out=w593:refnum<visa-resource-name>, error out=w594:errorcluster)  [unwired: 1 out]
              n221 = Wait Until Next ms Multiple(millisecond multiple=u32 5) -> ()  [unwired: 1 out]
            }
            n222 = disable-structure shown="Disabled" {
              disable-tunnel: [w575 w591] -> w561
              disable-tunnel: [w574 w592] -> w560
              disable-tunnel: w558 -> [w569 w592]
              disable-tunnel: w557 -> [w565 w591]
              frame Disabled {
                n223 = call "Timer2.vi"("error in (no error)"=w565, "Reset"=TRUE) -> ("error out"=w564:errorcluster)  [unwired: 7 in, 2 out]
                n224 = while {
                  tunnel: w569 -> [w581]
                  tunnel: [w581] -> w568
                  tunnel: [w579] -> w567
                  tunnel: w564 -> [w580]
                  stop <- w578 stop-if-true
                  n225 = call "Timer2.vi"("error in (no error)"=w580, "Time Target (s)"=0.25, "Pause"=TRUE) -> ("error out"=w579:errorcluster, "Time has Elapsed"=w578:bool)  [unwired: 6 in, 1 out]
                }
                n226 = property class="Instr"(reference=w568, error in=w567) -> (reference out=w572:refnum<visa-resource-name>, error out=w571:errorcluster, "Bytes at Port"=w570:u32)
                n227 = for {
                  N: w570 -> [_]
                  tunnel: w571 -> [w589]
                  tunnel: w572 -> [w588]
                  shift-right: [w583] -> _
                  shift-left: "" -> [w587]
                  tunnel: [w586] -> w575
                  tunnel: [w585] -> w574
                  n228 = VISA Read(VISA resource name=w588, byte count=u32 1, error in (no error)=w589) -> (VISA resource name out=w585:refnum<visa-resource-name>, read buffer=w582:string, error out=w586:errorcluster)  [unwired: 1 out]
                  n229 = Concatenate Strings(w587, w582) -> (w583:string)
                  n230 = Wait Until Next ms Multiple(millisecond multiple=u32 5) -> ()  [unwired: 1 out]
                }
              }
              frame Enabled {
              }
            }
          }
          frame "Dorsales" {
            n231 = Unbundle By Name(w604) -> ("Dorsales"=w602:i32)
            n232 = To Unsigned Byte Integer(number=w602) -> (unsigned 8bit integer=w603:u8)
            n233 = Build Array(w603) -> (w608:u8[])
            n234 = Byte Array To String(unsigned byte array=w608) -> (string=w606:string)
            n235 = Concatenate Strings("6", w606) -> (w605:string)
            n236 = String Length(string=w605) -> (length=w611:i32)
            n237 = for {
              N: w611 -> [_]
              tunnel: w614 -> [w653]
              tunnel: w615 -> [w652]
              tunnel: w605 -> [w649]
              tunnel: [w646] -> w609
              tunnel: [w645] -> w610
              i -> [w647]
              n238 = String Subset(string=w649, offset (0)=w647, length (rest)=1 ("length (rest)")) -> (substring=w650:string)
              n239 = VISA Write(VISA resource name=w652, write buffer=w650, error in (no error)=w653) -> (VISA resource name out=w645:refnum<visa-resource-name>, error out=w646:errorcluster)  [unwired: 1 out]
              n240 = Wait Until Next ms Multiple(millisecond multiple=u32 5) -> ()  [unwired: 1 out]
            }
            n241 = disable-structure shown="Disabled" {
              disable-tunnel: [w627 w643] -> w613
              disable-tunnel: [w626 w644] -> w612
              disable-tunnel: w610 -> [w621 w644]
              disable-tunnel: w609 -> [w617 w643]
              frame Disabled {
                n242 = call "Timer2.vi"("error in (no error)"=w617, "Reset"=TRUE) -> ("error out"=w616:errorcluster)  [unwired: 7 in, 2 out]
                n243 = while {
                  tunnel: w621 -> [w633]
                  tunnel: [w633] -> w620
                  tunnel: [w631] -> w619
                  tunnel: w616 -> [w632]
                  stop <- w630 stop-if-true
                  n244 = call "Timer2.vi"("error in (no error)"=w632, "Time Target (s)"=0.25, "Pause"=TRUE) -> ("error out"=w631:errorcluster, "Time has Elapsed"=w630:bool)  [unwired: 6 in, 1 out]
                }
                n245 = property class="Instr"(reference=w620, error in=w619) -> (reference out=w624:refnum<visa-resource-name>, error out=w623:errorcluster, "Bytes at Port"=w622:u32)
                n246 = for {
                  N: w622 -> [_]
                  tunnel: w623 -> [w641]
                  tunnel: w624 -> [w640]
                  shift-right: [w635] -> _
                  shift-left: "" -> [w639]
                  tunnel: [w638] -> w627
                  tunnel: [w637] -> w626
                  n247 = VISA Read(VISA resource name=w640, byte count=u32 1, error in (no error)=w641) -> (VISA resource name out=w637:refnum<visa-resource-name>, read buffer=w634:string, error out=w638:errorcluster)  [unwired: 1 out]
                  n248 = Concatenate Strings(w639, w634) -> (w635:string)
                  n249 = Wait Until Next ms Multiple(millisecond multiple=u32 5) -> ()  [unwired: 1 out]
                }
              }
              frame Enabled {
              }
            }
          }
          frame "Trapecio" {
            n250 = Unbundle By Name(w656) -> ("Trapecio"=w654:i32)
            n251 = To Unsigned Byte Integer(number=w654) -> (unsigned 8bit integer=w655:u8)
            n252 = Build Array(w655) -> (w660:u8[])
            n253 = Byte Array To String(unsigned byte array=w660) -> (string=w658:string)
            n254 = Concatenate Strings("7", w658) -> (w657:string)
            n255 = String Length(string=w657) -> (length=w663:i32)
            n256 = for {
              N: w663 -> [_]
              tunnel: w666 -> [w705]
              tunnel: w667 -> [w704]
              tunnel: w657 -> [w701]
              tunnel: [w698] -> w661
              tunnel: [w697] -> w662
              i -> [w699]
              n257 = String Subset(string=w701, offset (0)=w699, length (rest)=1 ("length (rest)")) -> (substring=w702:string)
              n258 = VISA Write(VISA resource name=w704, write buffer=w702, error in (no error)=w705) -> (VISA resource name out=w697:refnum<visa-resource-name>, error out=w698:errorcluster)  [unwired: 1 out]
              n259 = Wait Until Next ms Multiple(millisecond multiple=u32 5) -> ()  [unwired: 1 out]
            }
            n260 = disable-structure shown="Disabled" {
              disable-tunnel: [w679 w695] -> w665
              disable-tunnel: [w678 w696] -> w664
              disable-tunnel: w662 -> [w673 w696]
              disable-tunnel: w661 -> [w669 w695]
              frame Disabled {
                n261 = call "Timer2.vi"("error in (no error)"=w669, "Reset"=TRUE) -> ("error out"=w668:errorcluster)  [unwired: 7 in, 2 out]
                n262 = while {
                  tunnel: w673 -> [w685]
                  tunnel: [w685] -> w672
                  tunnel: [w683] -> w671
                  tunnel: w668 -> [w684]
                  stop <- w682 stop-if-true
                  n263 = call "Timer2.vi"("error in (no error)"=w684, "Time Target (s)"=0.25, "Pause"=TRUE) -> ("error out"=w683:errorcluster, "Time has Elapsed"=w682:bool)  [unwired: 6 in, 1 out]
                }
                n264 = property class="Instr"(reference=w672, error in=w671) -> (reference out=w676:refnum<visa-resource-name>, error out=w675:errorcluster, "Bytes at Port"=w674:u32)
                n265 = for {
                  N: w674 -> [_]
                  tunnel: w675 -> [w693]
                  tunnel: w676 -> [w692]
                  shift-right: [w687] -> _
                  shift-left: "" -> [w691]
                  tunnel: [w690] -> w679
                  tunnel: [w689] -> w678
                  n266 = VISA Read(VISA resource name=w692, byte count=u32 1, error in (no error)=w693) -> (VISA resource name out=w689:refnum<visa-resource-name>, read buffer=w686:string, error out=w690:errorcluster)  [unwired: 1 out]
                  n267 = Concatenate Strings(w691, w686) -> (w687:string)
                  n268 = Wait Until Next ms Multiple(millisecond multiple=u32 5) -> ()  [unwired: 1 out]
                }
              }
              frame Enabled {
              }
            }
          }
          frame "Pectorales" {
            n269 = Unbundle By Name(w708) -> ("Pectorales"=w706:i32)
            n270 = To Unsigned Byte Integer(number=w706) -> (unsigned 8bit integer=w707:u8)
            n271 = Build Array(w707) -> (w712:u8[])
            n272 = Byte Array To String(unsigned byte array=w712) -> (string=w710:string)
            n273 = Concatenate Strings("8", w710) -> (w709:string)
            n274 = String Length(string=w709) -> (length=w715:i32)
            n275 = for {
              N: w715 -> [_]
              tunnel: w718 -> [w757]
              tunnel: w719 -> [w756]
              tunnel: w709 -> [w753]
              tunnel: [w750] -> w713
              tunnel: [w749] -> w714
              i -> [w751]
              n276 = String Subset(string=w753, offset (0)=w751, length (rest)=1 ("length (rest)")) -> (substring=w754:string)
              n277 = VISA Write(VISA resource name=w756, write buffer=w754, error in (no error)=w757) -> (VISA resource name out=w749:refnum<visa-resource-name>, error out=w750:errorcluster)  [unwired: 1 out]
              n278 = Wait Until Next ms Multiple(millisecond multiple=u32 5) -> ()  [unwired: 1 out]
            }
            n279 = disable-structure shown="Disabled" {
              disable-tunnel: [w731 w747] -> w717
              disable-tunnel: [w730 w748] -> w716
              disable-tunnel: w714 -> [w725 w748]
              disable-tunnel: w713 -> [w721 w747]
              frame Disabled {
                n280 = call "Timer2.vi"("error in (no error)"=w721, "Reset"=TRUE) -> ("error out"=w720:errorcluster)  [unwired: 7 in, 2 out]
                n281 = while {
                  tunnel: w725 -> [w737]
                  tunnel: [w737] -> w724
                  tunnel: [w735] -> w723
                  tunnel: w720 -> [w736]
                  stop <- w734 stop-if-true
                  n282 = call "Timer2.vi"("error in (no error)"=w736, "Time Target (s)"=0.25, "Pause"=TRUE) -> ("error out"=w735:errorcluster, "Time has Elapsed"=w734:bool)  [unwired: 6 in, 1 out]
                }
                n283 = property class="Instr"(reference=w724, error in=w723) -> (reference out=w728:refnum<visa-resource-name>, error out=w727:errorcluster, "Bytes at Port"=w726:u32)
                n284 = for {
                  N: w726 -> [_]
                  tunnel: w727 -> [w745]
                  tunnel: w728 -> [w744]
                  shift-right: [w739] -> _
                  shift-left: "" -> [w743]
                  tunnel: [w742] -> w731
                  tunnel: [w741] -> w730
                  n285 = VISA Read(VISA resource name=w744, byte count=u32 1, error in (no error)=w745) -> (VISA resource name out=w741:refnum<visa-resource-name>, read buffer=w738:string, error out=w742:errorcluster)  [unwired: 1 out]
                  n286 = Concatenate Strings(w743, w738) -> (w739:string)
                  n287 = Wait Until Next ms Multiple(millisecond multiple=u32 5) -> ()  [unwired: 1 out]
                }
              }
              frame Enabled {
              }
            }
          }
          frame "Biceps" {
            n288 = Unbundle By Name(w760) -> ("Biceps"=w758:i32)
            n289 = To Unsigned Byte Integer(number=w758) -> (unsigned 8bit integer=w759:u8)
            n290 = Build Array(w759) -> (w764:u8[])
            n291 = Byte Array To String(unsigned byte array=w764) -> (string=w762:string)
            n292 = Concatenate Strings("9", w762) -> (w761:string)
            n293 = String Length(string=w761) -> (length=w767:i32)
            n294 = for {
              N: w767 -> [_]
              tunnel: w770 -> [w809]
              tunnel: w771 -> [w808]
              tunnel: w761 -> [w805]
              tunnel: [w802] -> w765
              tunnel: [w801] -> w766
              i -> [w803]
              n295 = String Subset(string=w805, offset (0)=w803, length (rest)=1 ("length (rest)")) -> (substring=w806:string)
              n296 = VISA Write(VISA resource name=w808, write buffer=w806, error in (no error)=w809) -> (VISA resource name out=w801:refnum<visa-resource-name>, error out=w802:errorcluster)  [unwired: 1 out]
              n297 = Wait Until Next ms Multiple(millisecond multiple=u32 5) -> ()  [unwired: 1 out]
            }
            n298 = disable-structure shown="Disabled" {
              disable-tunnel: [w783 w799] -> w769
              disable-tunnel: [w782 w800] -> w768
              disable-tunnel: w766 -> [w777 w800]
              disable-tunnel: w765 -> [w773 w799]
              frame Disabled {
                n299 = call "Timer2.vi"("error in (no error)"=w773, "Reset"=TRUE) -> ("error out"=w772:errorcluster)  [unwired: 7 in, 2 out]
                n300 = while {
                  tunnel: w777 -> [w789]
                  tunnel: [w789] -> w776
                  tunnel: [w787] -> w775
                  tunnel: w772 -> [w788]
                  stop <- w786 stop-if-true
                  n301 = call "Timer2.vi"("error in (no error)"=w788, "Time Target (s)"=0.25, "Pause"=TRUE) -> ("error out"=w787:errorcluster, "Time has Elapsed"=w786:bool)  [unwired: 6 in, 1 out]
                }
                n302 = property class="Instr"(reference=w776, error in=w775) -> (reference out=w780:refnum<visa-resource-name>, error out=w779:errorcluster, "Bytes at Port"=w778:u32)
                n303 = for {
                  N: w778 -> [_]
                  tunnel: w779 -> [w797]
                  tunnel: w780 -> [w796]
                  shift-right: [w791] -> _
                  shift-left: "" -> [w795]
                  tunnel: [w794] -> w783
                  tunnel: [w793] -> w782
                  n304 = VISA Read(VISA resource name=w796, byte count=u32 1, error in (no error)=w797) -> (VISA resource name out=w793:refnum<visa-resource-name>, read buffer=w790:string, error out=w794:errorcluster)  [unwired: 1 out]
                  n305 = Concatenate Strings(w795, w790) -> (w791:string)
                  n306 = Wait Until Next ms Multiple(millisecond multiple=u32 5) -> ()  [unwired: 1 out]
                }
              }
              frame Enabled {
              }
            }
          }
          frame "Opcional" {
            n307 = Unbundle By Name(w812) -> ("Opcional"=w810:i32)
            n308 = To Unsigned Byte Integer(number=w810) -> (unsigned 8bit integer=w811:u8)
            n309 = Build Array(w811) -> (w816:u8[])
            n310 = Byte Array To String(unsigned byte array=w816) -> (string=w814:string)
            n311 = Concatenate Strings("10", w814) -> (w813:string)
            n312 = String Length(string=w813) -> (length=w819:i32)
            n313 = for {
              N: w819 -> [_]
              tunnel: w822 -> [w861]
              tunnel: w823 -> [w860]
              tunnel: w813 -> [w857]
              tunnel: [w854] -> w817
              tunnel: [w853] -> w818
              i -> [w855]
              n314 = String Subset(string=w857, offset (0)=w855, length (rest)=1 ("length (rest)")) -> (substring=w858:string)
              n315 = VISA Write(VISA resource name=w860, write buffer=w858, error in (no error)=w861) -> (VISA resource name out=w853:refnum<visa-resource-name>, error out=w854:errorcluster)  [unwired: 1 out]
              n316 = Wait Until Next ms Multiple(millisecond multiple=u32 5) -> ()  [unwired: 1 out]
            }
            n317 = disable-structure shown="Disabled" {
              disable-tunnel: [w835 w851] -> w821
              disable-tunnel: [w834 w852] -> w820
              disable-tunnel: w818 -> [w829 w852]
              disable-tunnel: w817 -> [w825 w851]
              frame Disabled {
                n318 = call "Timer2.vi"("error in (no error)"=w825, "Reset"=TRUE) -> ("error out"=w824:errorcluster)  [unwired: 7 in, 2 out]
                n319 = while {
                  tunnel: w829 -> [w841]
                  tunnel: [w841] -> w828
                  tunnel: [w839] -> w827
                  tunnel: w824 -> [w840]
                  stop <- w838 stop-if-true
                  n320 = call "Timer2.vi"("error in (no error)"=w840, "Time Target (s)"=0.25, "Pause"=TRUE) -> ("error out"=w839:errorcluster, "Time has Elapsed"=w838:bool)  [unwired: 6 in, 1 out]
                }
                n321 = property class="Instr"(reference=w828, error in=w827) -> (reference out=w832:refnum<visa-resource-name>, error out=w831:errorcluster, "Bytes at Port"=w830:u32)
                n322 = for {
                  N: w830 -> [_]
                  tunnel: w831 -> [w849]
                  tunnel: w832 -> [w848]
                  shift-right: [w843] -> _
                  shift-left: "" -> [w847]
                  tunnel: [w846] -> w835
                  tunnel: [w845] -> w834
                  n323 = VISA Read(VISA resource name=w848, byte count=u32 1, error in (no error)=w849) -> (VISA resource name out=w845:refnum<visa-resource-name>, read buffer=w842:string, error out=w846:errorcluster)  [unwired: 1 out]
                  n324 = Concatenate Strings(w847, w842) -> (w843:string)
                  n325 = Wait Until Next ms Multiple(millisecond multiple=u32 5) -> ()  [unwired: 1 out]
                }
              }
              frame Enabled {
              }
            }
          }
        }
      }
      frame Error {
        # "Return true in any case that should stop the loop."
      }
    }
  }
  n326 = while {
    tunnel: w15 -> [_]
    tunnel: w8 -> [w869]
    shift-right: [w867] -> _
    shift-left: w10 -> [w868]
    shift-right: [w865] -> w2
    shift-left: w3 -> [w866]
    stop <- w871 stop-if-true
    n327 = event shown="[0] Timeout" {
      selector: _ -> [_ _ _ _ _ _ _ _ _ _ _ _ _ _ _ _ _ _ _ _]
      dyn-events: _ -> [_ _ _ _ _ _ _ _ _ _ _ _ _ _ _ _ _ _ _ _]
      timeout: 300 -> [_ _ _ _ _ _ _ _ _ _ _ _ _ _ _ _ _ _ _ _]
      tunnel: [w877 FALSE FALSE FALSE FALSE FALSE FALSE FALSE FALSE FALSE FALSE _ _ _ TRUE ("Stop") FALSE ("Stop") FALSE ("Stop") FALSE ("Stop") FALSE ("Stop") FALSE ("Stop")] -> w871
      tunnel: w869 -> [w875 _ _ _ _ _ _ _ _ _ _ w1246 w1396 w1511 _ _ _ w1649 w1701 w1707]
      tunnel: w868 -> [w873 w1007 w1032 w1058 w1083 w1108 w1133 w1158 w1183 w1208 w1233 w1249 w1398 w1515 w1588 w1591 w1620 w1629 w1702 w1711]
      tunnel: [w872 w1008 w1033 w1057 w1082 w1107 w1132 w1157 w1182 w1207 w1232 w1250 w1399 w1516 w1586 w1590 w1620 w1634 w1653 w1710] -> w867
      tunnel: w866 -> [w874 _ _ _ _ _ _ _ _ _ _ w1247 w1395 w1512 _ _ _ w1648 w1700 w1706]
      tunnel: [_ _ _ _ _ _ _ _ _ _ _ _ _ _ _ _ _ w1636 _ w1705] -> w865
      event Timeout {
        n328 = event-data() -> ()  [unwired: 1 in, 3 out]
        n329 = Unbundle By Name(w873) -> ("Label"=w893:string, "Cuadriceps"=w892:i32, "Isquiotibiales"=w891:i32, "Gluteos"=w890:i32, "Abdomen"=w889:i32, "Lumbares"=w888:i32, "Dorsales"=w887:i32, "Trapecio"=w886:i32, "Pectorales"=w885:i32, "Biceps"=w884:i32, "Opcional"=w883:i32, "Master"=w879:i32, "Slider"=w878:i32)
        n330 = Unbundle By Name(w873) -> ("Impulso"=w881:i32, "Tiempo"=w880:i32)
        n331 = Format Date/Time String() -> (date/time string=→"date/time string":string)  [unwired: 3 in]
        n332 = local read "Start?"() -> (w894:bool)
        n333 = case shown="\"Cuadriceps\"" w893 {
          selector: w893 -> [w943 w948 w953 w958 w963 w968 w973 w978 w983 w988 w993 w995]
          tunnel: [w943 w948 w953 w958 w963 w968 w973 w978 w983 w988 w993 w995] -> _
          tunnel: [w939 w944 w949 w954 w959 w964 w969 w974 w979 w984 w989 w994] -> w882
          tunnel: w892 -> [w939 _ _ _ _ _ _ _ _ _ _ _]
          tunnel: w891 -> [_ w944 _ _ _ _ _ _ _ _ _ _]
          tunnel: w890 -> [_ _ w949 _ _ _ _ _ _ _ _ _]
          tunnel: w889 -> [_ _ _ w954 _ _ _ _ _ _ _ _]
          tunnel: w888 -> [_ _ _ _ w959 _ _ _ _ _ _ _]
          tunnel: w887 -> [_ _ _ _ _ w964 _ _ _ _ _ _]
          tunnel: w886 -> [_ _ _ _ _ _ w969 _ _ _ _ _]
          tunnel: w885 -> [_ _ _ _ _ _ _ w974 _ _ _ _]
          tunnel: w884 -> [_ _ _ _ _ _ _ _ w979 _ _ _]
          tunnel: w883 -> [_ _ _ _ _ _ _ _ _ w984 _ _]
          tunnel: w879 -> [_ _ _ _ _ _ _ _ _ _ w989 _]
          tunnel: w878 -> [_ _ _ _ _ _ _ _ _ _ _ w994]
          frame "Cuadriceps" {
            n334 = Number To Decimal String(number=w939) -> (decimal integer string=w942:string)  [unwired: 1 in]
            n335 = Concatenate Strings(w942, "%" ("string")) -> (→"Cuadríceps %":string)
          }
          frame "Isquiotibiales" {
            n336 = Number To Decimal String(number=w944) -> (decimal integer string=w947:string)  [unwired: 1 in]
            n337 = Concatenate Strings(w947, "%" ("string")) -> (→"Isquiotibiales %":string)
          }
          frame "Gluteos" {
            n338 = Number To Decimal String(number=w949) -> (decimal integer string=w952:string)  [unwired: 1 in]
            n339 = Concatenate Strings(w952, "%" ("string")) -> (→"Gluteos %":string)
          }
          frame "Abdomen" {
            n340 = Number To Decimal String(number=w954) -> (decimal integer string=w957:string)  [unwired: 1 in]
            n341 = Concatenate Strings(w957, "%" ("string")) -> (→"Abdomen %":string)
          }
          frame "Lumbares" {
            n342 = Number To Decimal String(number=w959) -> (decimal integer string=w962:string)  [unwired: 1 in]
            n343 = Concatenate Strings(w962, "%" ("string")) -> (→"Lumbares %":string)
          }
          frame "Dorsales" {
            n344 = Number To Decimal String(number=w964) -> (decimal integer string=w967:string)  [unwired: 1 in]
            n345 = Concatenate Strings(w967, "%" ("string")) -> (→"Dorsales %":string)
          }
          frame "Trapecio" {
            n346 = Number To Decimal String(number=w969) -> (decimal integer string=w972:string)  [unwired: 1 in]
            n347 = Concatenate Strings(w972, "%" ("string")) -> (→"Trapecio %":string)
          }
          frame "Pectorales" {
            n348 = Number To Decimal String(number=w974) -> (decimal integer string=w977:string)  [unwired: 1 in]
            n349 = Concatenate Strings(w977, "%" ("string")) -> (→"Pectorales %":string)
          }
          frame "Biceps" {
            n350 = Number To Decimal String(number=w979) -> (decimal integer string=w982:string)  [unwired: 1 in]
            n351 = Concatenate Strings(w982, "%" ("string")) -> (→"Biceps %":string)
          }
          frame "Opcional" {
            n352 = Number To Decimal String(number=w984) -> (decimal integer string=w987:string)  [unwired: 1 in]
            n353 = Concatenate Strings(w987, "%" ("string")) -> (→"Opcional %":string)
          }
          frame "Master" {
            n354 = Number To Decimal String(number=w989) -> (decimal integer string=w992:string)  [unwired: 1 in]
            n355 = Concatenate Strings(w992, "%" ("string")) -> (→"Master Ind":string)
          }
          frame "Inicio", Default {
          }
        }
        "Horizontal Graduated Bar" <- w882
        n356 = case shown="True" w894 {
          tunnel: w880 -> [_ w911]
          tunnel: w881 -> [_ w910]
          tunnel: [_ w900] -> w877
          tunnel: w873 -> [_ w909]
          tunnel: w875 -> [_ w905]
          tunnel: w874 -> [_ w904]
          tunnel: w873 -> [w895 w903]
          tunnel: [w895 w902] -> w872
          frame False {
            n357 = property on="Start" class="Bool (strict)"("BoolText.Text"="Start / Inicio" ("Boolean Text.Text")) -> ()  [unwired: 2 in, 2 out]
            n358 = flat-sequence {
              tunnel: [w897] -> _
              frame #0 {
                w897 = FALSE ("Visible")
                n359 = property on="Tiempo Restante" class="Str"("Visible"=w897) -> (error out=w898:errorcluster)  [unwired: 2 in, 1 out]
                n360 = property on="Tiempo Transcurrido" class="Str"(error in=w898, "Visible"=w897) -> ()  [unwired: 1 in, 2 out]
              }
            }
          }
          frame True {
            n361 = Unbundle By Name(w909) -> ("Label"=w906:string, "Impulso"=w908:i32, "Ruptura"=w907:i32)
            n362 = Number To Decimal String(number=w910) -> (decimal integer string=→"Hola":string)  [unwired: 1 in]
            n363 = Multiply(x=w911, y=60) -> (x*y=w901:i32)
            n364 = property on="Start" class="Bool (strict)"("BoolText.Text"="Stop / Parar" ("Boolean Text.Text")) -> ()  [unwired: 2 in, 2 out]
            n365 = call "Elapsed Time"("Time Target (s)"=w901) -> ("Elapsed Time (s)"=w899:dbl, "Time has Elapsed"=w900:bool)  [unwired: 11 in, 6 out]
            n366 = Subtract(x=w901, y=w899) -> (x-y=w918:dbl)
            n367 = To Time Stamp(1:w918) -> (0:w915:timestamp)
            n368 = To Time Stamp(1:w899) -> (0:w919:timestamp)
            n369 = Format Date/Time String(time format string (%c)="%M : %S", seconds (now)=w915) -> (date/time string=→"Tiempo Restante":string)  [unwired: 1 in]
            n370 = case shown="\"Encender\"" w906 {
              tunnel: w908 -> [w929 w936 _]
              tunnel: w907 -> [w928 w935 _]
              tunnel: w905 -> [w927 w934 _]
              tunnel: w904 -> [w926 w933 _]
              tunnel: w903 -> [w925 w932 w938]
              tunnel: [w924 w931 w938] -> w902
              frame "Start" {
                n371 = Bundle By Name(cluster=w925, "Label"="Encender", "Impulso"=w929, "Ruptura"=w928) -> (w924:T1)
                n372 = Enqueue Element(queue=w927, element=w924, error in (no error)=w926) -> ()  [unwired: 1 in, 3 out]
              }
              frame "Encender" {
                n373 = Bundle By Name(cluster=w932, "Label"="Encender", "Impulso"=w936, "Ruptura"=w935) -> (w931:T1)
                n374 = Enqueue Element(queue=w934, element=w931, error in (no error)=w933) -> ()  [unwired: 1 in, 3 out]
              }
              frame "Inicio", Default {
              }
            }
            n375 = Format Date/Time String(time format string (%c)="%M : %S", seconds (now)=w919) -> (date/time string=→"Tiempo Transcurrido":string)  [unwired: 1 in]
            n376 = flat-sequence {
              tunnel: [w922] -> _
              frame #0 {
                w922 = TRUE ("Visible")
                n377 = property on="Tiempo Restante" class="Str"("Visible"=w922) -> (error out=w923:errorcluster)  [unwired: 2 in, 1 out]
                n378 = property on="Tiempo Transcurrido" class="Str"(error in=w923, "Visible"=w922) -> ()  [unwired: 1 in, 2 out]
              }
            }
          }
        }
        n379 = local write "Slider"(w882) -> ()
      }
      event "Cuadriceps Bool": Value Change {
        n380 = event-data() -> ()  [unwired: 1 in, 6 out]
        n381 = Bundle By Name(cluster=cluster{"Color Box":u32, "Color Box 2":u32} {"Color Box"=12369084, "Color Box 2"=12369084}, "Color Box"=u32 16711680 ("Color Box 2")) -> (w1017:cluster{"Color Box":u32, "Color Box 2":u32})
        n382 = Bundle By Name(cluster=cluster{"Color Box":u32, "Color Box 2":u32} {"Color Box"=12369084, "Color Box 2"=12369084}, "Color Box"=u32 12369084 ("Color Box 2")) -> (w1012:cluster{"Color Box":u32, "Color Box 2":u32})
        n383 = Bundle By Name(cluster=w1007, "Label"="Cuadriceps" ("Message")) -> (w1008:T1)
        n384 = property on="Master" class="Bool (strict)"() -> (error out=w997:errorcluster, "Colors [4]"=w1000:cluster{u32, u32}[])  [unwired: 2 in, 1 out]
        n385 = Insert Into Array(array=cluster{u32, u32}[] [] ("Colors [4]"), new element=w1017) -> (w1016:cluster{u32, u32}[])  [unwired: 1 in]
        n386 = Insert Into Array(array=cluster{u32, u32}[] [] ("Colors [4]"), new element=w1012) -> (w1010:cluster{u32, u32}[])  [unwired: 1 in]
        n387 = Index Array(array=w1000) -> (element=w1006:cluster{u32, u32})  [unwired: 1 in]
        n388 = property on="Cuadriceps Bool" class="Bool"("Colors [4]"=w1016) -> ()  [unwired: 2 in, 2 out]
        n389 = Unbundle(w1006) -> (w1002:u32)  [unwired: 1 out]
        n390 = property on="Abdomen Bool" class="Bool"("Colors [4]"=w1010) -> ()  [unwired: 2 in, 2 out]
        n391 = property on="Lumbares Bool" class="Bool"("Colors [4]"=w1010) -> ()  [unwired: 2 in, 2 out]
        n392 = property on="Gluteos Bool" class="Bool"("Colors [4]"=w1010) -> ()  [unwired: 2 in, 2 out]
        n393 = property on="Isquiotibiales Bool" class="Bool"("Colors [4]"=w1010) -> ()  [unwired: 2 in, 2 out]
        n394 = Bundle(w1002, "Boolean Text.Text Colors:Text Color"=u32 40709) -> (w1005:T2)  [unwired: 1 in]
        n395 = property on="Pectorales Bool" class="Bool"("Colors [4]"=w1010) -> ()  [unwired: 2 in, 2 out]
        n396 = property on="Dorsales Bool" class="Bool"("Colors [4]"=w1010) -> ()  [unwired: 2 in, 2 out]
        n397 = property on="Trapecio Bool" class="Bool"("Colors [4]"=w1010) -> ()  [unwired: 2 in, 2 out]
        n398 = property on="Opcional Bool" class="Bool"("Colors [4]"=w1010) -> ()  [unwired: 2 in, 2 out]
        n399 = property on="Biceps Bool" class="Bool"("Colors [4]"=w1010) -> ()  [unwired: 2 in, 2 out]
        n400 = Replace Array Subset(array=w1000, new element=w1005, index=0) -> (w999:cluster{u32, u32}[])
        n401 = property on="Master" class="Bool (strict)"(error in=w997, "Colors [4]"=w999) -> (error out=w998:errorcluster)  [unwired: 1 in, 1 out]
        n402 = local write "Master"(FALSE ("Master")) -> ()
        n403 = property on="Master" class="Bool (strict)"(error in=w998, "BoolText.TextColor"=u32 16448250 ("Boolean Text.Text Colors:Text Color")) -> ()  [unwired: 1 in, 2 out]
      }
      event "Isquiotibiales Bool": Value Change {
        n404 = event-data() -> ()  [unwired: 1 in, 6 out]
        n405 = Bundle By Name(cluster=cluster{"Color Box":u32, "Color Box 2":u32} {"Color Box"=12369084, "Color Box 2"=12369084}, "Color Box"=u32 16711680 ("Color Box 2")) -> (w1042:cluster{"Color Box":u32, "Color Box 2":u32})
        n406 = Bundle By Name(cluster=cluster{"Color Box":u32, "Color Box 2":u32} {"Color Box"=12369084, "Color Box 2"=12369084}, "Color Box"=u32 12369084 ("Color Box 2")) -> (w1038:cluster{"Color Box":u32, "Color Box 2":u32})
        n407 = Bundle By Name(cluster=w1032, "Label"="Isquiotibiales" ("Message")) -> (w1033:T1)
        n408 = property on="Master" class="Bool (strict)"() -> (error out=w1022:errorcluster, "Colors [4]"=w1025:cluster{u32, u32}[])  [unwired: 2 in, 1 out]
        n409 = Insert Into Array(array=cluster{u32, u32}[] [] ("Colors [4]"), new element=w1042) -> (w1036:cluster{u32, u32}[])  [unwired: 1 in]
        n410 = Insert Into Array(array=cluster{u32, u32}[] [] ("Colors [4]"), new element=w1038) -> (w1035:cluster{u32, u32}[])  [unwired: 1 in]
        n411 = local write "Master"(FALSE ("Master")) -> ()
        n412 = Index Array(array=w1025) -> (element=w1031:cluster{u32, u32})  [unwired: 1 in]
        n413 = property on="Isquiotibiales Bool" class="Bool"("Colors [4]"=w1036) -> ()  [unwired: 2 in, 2 out]
        n414 = property on="Abdomen Bool" class="Bool"("Colors [4]"=w1035) -> ()  [unwired: 2 in, 2 out]
        n415 = property on="Lumbares Bool" class="Bool"("Colors [4]"=w1035) -> ()  [unwired: 2 in, 2 out]
        n416 = property on="Gluteos Bool" class="Bool"("Colors [4]"=w1035) -> ()  [unwired: 2 in, 2 out]
        n417 = property on="Cuadriceps Bool" class="Bool"("Colors [4]"=w1035) -> ()  [unwired: 2 in, 2 out]
        n418 = Unbundle(w1031) -> (w1027:u32)  [unwired: 1 out]
        n419 = Bundle(w1027, "Boolean Text.Text Colors:Text Color"=u32 40709) -> (w1030:T2)  [unwired: 1 in]
        n420 = property on="Pectorales Bool" class="Bool"("Colors [4]"=w1035) -> ()  [unwired: 2 in, 2 out]
        n421 = property on="Dorsales Bool" class="Bool"("Colors [4]"=w1035) -> ()  [unwired: 2 in, 2 out]
        n422 = property on="Trapecio Bool" class="Bool"("Colors [4]"=w1035) -> ()  [unwired: 2 in, 2 out]
        n423 = property on="Opcional Bool" class="Bool"("Colors [4]"=w1035) -> ()  [unwired: 2 in, 2 out]
        n424 = property on="Biceps Bool" class="Bool"("Colors [4]"=w1035) -> ()  [unwired: 2 in, 2 out]
        n425 = Replace Array Subset(array=w1025, new element=w1030, index=0) -> (w1024:cluster{u32, u32}[])
        n426 = property on="Master" class="Bool (strict)"(error in=w1022, "Colors [4]"=w1024) -> (error out=w1023:errorcluster)  [unwired: 1 in, 1 out]
        n427 = property on="Master" class="Bool (strict)"(error in=w1023, "BoolText.TextColor"=u32 16448250 ("Boolean Text.Text Colors:Text Color")) -> ()  [unwired: 1 in, 2 out]
      }
      event "Gluteos Bool": Value Change {
        n428 = event-data() -> ()  [unwired: 1 in, 6 out]
        n429 = Bundle By Name(cluster=cluster{"Color Box":u32, "Color Box 2":u32} {"Color Box"=12369084, "Color Box 2"=12369084}, "Color Box"=u32 16711680 ("Color Box 2")) -> (w1067:cluster{"Color Box":u32, "Color Box 2":u32})
        n430 = Bundle By Name(cluster=cluster{"Color Box":u32, "Color Box 2":u32} {"Color Box"=12369084, "Color Box 2"=12369084}, "Color Box"=u32 12369084 ("Color Box 2")) -> (w1063:cluster{"Color Box":u32, "Color Box 2":u32})
        n431 = Bundle By Name(cluster=w1058, "Label"="Gluteos" ("Message")) -> (w1057:T1)
        n432 = property on="Master" class="Bool (strict)"() -> (error out=w1047:errorcluster, "Colors [4]"=w1050:cluster{u32, u32}[])  [unwired: 2 in, 1 out]
        n433 = Insert Into Array(array=cluster{u32, u32}[] [] ("Colors [4]"), new element=w1067) -> (w1061:cluster{u32, u32}[])  [unwired: 1 in]
        n434 = Insert Into Array(array=cluster{u32, u32}[] [] ("Colors [4]"), new element=w1063) -> (w1060:cluster{u32, u32}[])  [unwired: 1 in]
        n435 = local write "Master"(FALSE ("Master")) -> ()
        n436 = property on="Gluteos Bool" class="Bool"("Colors [4]"=w1061) -> ()  [unwired: 2 in, 2 out]
        n437 = Index Array(array=w1050) -> (element=w1056:cluster{u32, u32})  [unwired: 1 in]
        n438 = property on="Abdomen Bool" class="Bool"("Colors [4]"=w1060) -> ()  [unwired: 2 in, 2 out]
        n439 = property on="Lumbares Bool" class="Bool"("Colors [4]"=w1060) -> ()  [unwired: 2 in, 2 out]
        n440 = property on="Isquiotibiales Bool" class="Bool"("Colors [4]"=w1060) -> ()  [unwired: 2 in, 2 out]
        n441 = property on="Cuadriceps Bool" class="Bool"("Colors [4]"=w1060) -> ()  [unwired: 2 in, 2 out]
        n442 = Unbundle(w1056) -> (w1052:u32)  [unwired: 1 out]
        n443 = property on="Pectorales Bool" class="Bool"("Colors [4]"=w1060) -> ()  [unwired: 2 in, 2 out]
        n444 = property on="Dorsales Bool" class="Bool"("Colors [4]"=w1060) -> ()  [unwired: 2 in, 2 out]
        n445 = property on="Trapecio Bool" class="Bool"("Colors [4]"=w1060) -> ()  [unwired: 2 in, 2 out]
        n446 = property on="Opcional Bool" class="Bool"("Colors [4]"=w1060) -> ()  [unwired: 2 in, 2 out]
        n447 = property on="Biceps Bool" class="Bool"("Colors [4]"=w1060) -> ()  [unwired: 2 in, 2 out]
        n448 = Bundle(w1052, "Boolean Text.Text Colors:Text Color"=u32 40709) -> (w1055:T2)  [unwired: 1 in]
        n449 = Replace Array Subset(array=w1050, new element=w1055, index=0) -> (w1049:cluster{u32, u32}[])
        n450 = property on="Master" class="Bool (strict)"(error in=w1047, "Colors [4]"=w1049) -> (error out=w1048:errorcluster)  [unwired: 1 in, 1 out]
        n451 = property on="Master" class="Bool (strict)"(error in=w1048, "BoolText.TextColor"=u32 16448250 ("Boolean Text.Text Colors:Text Color")) -> ()  [unwired: 1 in, 2 out]
      }
      event "Abdomen Bool": Value Change {
        n452 = event-data() -> ()  [unwired: 1 in, 6 out]
        n453 = Bundle By Name(cluster=cluster{"Color Box":u32, "Color Box 2":u32} {"Color Box"=12369084, "Color Box 2"=12369084}, "Color Box"=u32 16711680 ("Color Box 2")) -> (w1092:cluster{"Color Box":u32, "Color Box 2":u32})
        n454 = Bundle By Name(cluster=cluster{"Color Box":u32, "Color Box 2":u32} {"Color Box"=12369084, "Color Box 2"=12369084}, "Color Box"=u32 12369084 ("Color Box 2")) -> (w1088:cluster{"Color Box":u32, "Color Box 2":u32})
        n455 = Bundle By Name(cluster=w1083, "Label"="Abdomen" ("Message")) -> (w1082:T1)
        n456 = property on="Master" class="Bool (strict)"() -> (error out=w1072:errorcluster, "Colors [4]"=w1075:cluster{u32, u32}[])  [unwired: 2 in, 1 out]
        n457 = Insert Into Array(array=cluster{u32, u32}[] [] ("Colors [4]"), new element=w1092) -> (w1086:cluster{u32, u32}[])  [unwired: 1 in]
        n458 = Insert Into Array(array=cluster{u32, u32}[] [] ("Colors [4]"), new element=w1088) -> (w1085:cluster{u32, u32}[])  [unwired: 1 in]
        n459 = property on="Abdomen Bool" class="Bool"("Colors [4]"=w1086) -> ()  [unwired: 2 in, 2 out]
        n460 = Index Array(array=w1075) -> (element=w1081:cluster{u32, u32})  [unwired: 1 in]
        n461 = local write "Master"(FALSE ("Master")) -> ()
        n462 = property on="Gluteos Bool" class="Bool"("Colors [4]"=w1085) -> ()  [unwired: 2 in, 2 out]
        n463 = property on="Lumbares Bool" class="Bool"("Colors [4]"=w1085) -> ()  [unwired: 2 in, 2 out]
        n464 = property on="Isquiotibiales Bool" class="Bool"("Colors [4]"=w1085) -> ()  [unwired: 2 in, 2 out]
        n465 = property on="Cuadriceps Bool" class="Bool"("Colors [4]"=w1085) -> ()  [unwired: 2 in, 2 out]
        n466 = Unbundle(w1081) -> (w1077:u32)  [unwired: 1 out]
        n467 = property on="Pectorales Bool" class="Bool"("Colors [4]"=w1085) -> ()  [unwired: 2 in, 2 out]
        n468 = property on="Dorsales Bool" class="Bool"("Colors [4]"=w1085) -> ()  [unwired: 2 in, 2 out]
        n469 = property on="Trapecio Bool" class="Bool"("Colors [4]"=w1085) -> ()  [unwired: 2 in, 2 out]
        n470 = property on="Opcional Bool" class="Bool"("Colors [4]"=w1085) -> ()  [unwired: 2 in, 2 out]
        n471 = property on="Biceps Bool" class="Bool"("Colors [4]"=w1085) -> ()  [unwired: 2 in, 2 out]
        n472 = Bundle(w1077, "Boolean Text.Text Colors:Text Color"=u32 40709) -> (w1080:T2)  [unwired: 1 in]
        n473 = Replace Array Subset(array=w1075, new element=w1080, index=0) -> (w1074:cluster{u32, u32}[])
        n474 = property on="Master" class="Bool (strict)"(error in=w1072, "Colors [4]"=w1074) -> (error out=w1073:errorcluster)  [unwired: 1 in, 1 out]
        n475 = property on="Master" class="Bool (strict)"(error in=w1073, "BoolText.TextColor"=u32 16448250 ("Boolean Text.Text Colors:Text Color")) -> ()  [unwired: 1 in, 2 out]
      }
      event "Lumbares Bool": Value Change {
        n476 = event-data() -> ()  [unwired: 1 in, 6 out]
        n477 = Bundle By Name(cluster=cluster{"Color Box":u32, "Color Box 2":u32} {"Color Box"=12369084, "Color Box 2"=12369084}, "Color Box"=u32 16711680 ("Color Box 2")) -> (w1117:cluster{"Color Box":u32, "Color Box 2":u32})
        n478 = Bundle By Name(cluster=cluster{"Color Box":u32, "Color Box 2":u32} {"Color Box"=12369084, "Color Box 2"=12369084}, "Color Box"=u32 12369084 ("Color Box 2")) -> (w1113:cluster{"Color Box":u32, "Color Box 2":u32})
        n479 = property on="Master" class="Bool (strict)"() -> (error out=w1097:errorcluster, "Colors [4]"=w1100:cluster{u32, u32}[])  [unwired: 2 in, 1 out]
        n480 = Insert Into Array(array=cluster{u32, u32}[] [] ("Colors [4]"), new element=w1117) -> (w1111:cluster{u32, u32}[])  [unwired: 1 in]
        n481 = Insert Into Array(array=cluster{u32, u32}[] [] ("Colors [4]"), new element=w1113) -> (w1110:cluster{u32, u32}[])  [unwired: 1 in]
        n482 = Bundle By Name(cluster=w1108, "Label"="Lumbares" ("Message")) -> (w1107:T1)
        n483 = property on="Lumbares Bool" class="Bool"("Colors [4]"=w1111) -> ()  [unwired: 2 in, 2 out]
        n484 = local write "Master"(FALSE ("Master")) -> ()
        n485 = Index Array(array=w1100) -> (element=w1106:cluster{u32, u32})  [unwired: 1 in]
        n486 = property on="Gluteos Bool" class="Bool"("Colors [4]"=w1110) -> ()  [unwired: 2 in, 2 out]
        n487 = property on="Abdomen Bool" class="Bool"("Colors [4]"=w1110) -> ()  [unwired: 2 in, 2 out]
        n488 = property on="Isquiotibiales Bool" class="Bool"("Colors [4]"=w1110) -> ()  [unwired: 2 in, 2 out]
        n489 = property on="Cuadriceps Bool" class="Bool"("Colors [4]"=w1110) -> ()  [unwired: 2 in, 2 out]
        n490 = Unbundle(w1106) -> (w1102:u32)  [unwired: 1 out]
        n491 = property on="Pectorales Bool" class="Bool"("Colors [4]"=w1110) -> ()  [unwired: 2 in, 2 out]
        n492 = property on="Dorsales Bool" class="Bool"("Colors [4]"=w1110) -> ()  [unwired: 2 in, 2 out]
        n493 = property on="Trapecio Bool" class="Bool"("Colors [4]"=w1110) -> ()  [unwired: 2 in, 2 out]
        n494 = property on="Opcional Bool" class="Bool"("Colors [4]"=w1110) -> ()  [unwired: 2 in, 2 out]
        n495 = property on="Biceps Bool" class="Bool"("Colors [4]"=w1110) -> ()  [unwired: 2 in, 2 out]
        n496 = Bundle(w1102, "Boolean Text.Text Colors:Text Color"=u32 40709) -> (w1105:T2)  [unwired: 1 in]
        n497 = Replace Array Subset(array=w1100, new element=w1105, index=0) -> (w1099:cluster{u32, u32}[])
        n498 = property on="Master" class="Bool (strict)"(error in=w1097, "Colors [4]"=w1099) -> (error out=w1098:errorcluster)  [unwired: 1 in, 1 out]
        n499 = property on="Master" class="Bool (strict)"(error in=w1098, "BoolText.TextColor"=u32 16448250 ("Boolean Text.Text Colors:Text Color")) -> ()  [unwired: 1 in, 2 out]
      }
      event "Dorsales Bool": Value Change {
        n500 = event-data() -> ()  [unwired: 1 in, 6 out]
        n501 = Bundle By Name(cluster=cluster{"Color Box":u32, "Color Box 2":u32} {"Color Box"=12369084, "Color Box 2"=12369084}, "Color Box"=u32 16711680 ("Color Box 2")) -> (w1142:cluster{"Color Box":u32, "Color Box 2":u32})
        n502 = Bundle By Name(cluster=cluster{"Color Box":u32, "Color Box 2":u32} {"Color Box"=12369084, "Color Box 2"=12369084}, "Color Box"=u32 12369084 ("Color Box 2")) -> (w1138:cluster{"Color Box":u32, "Color Box 2":u32})
        n503 = property on="Master" class="Bool (strict)"() -> (error out=w1122:errorcluster, "Colors [4]"=w1125:cluster{u32, u32}[])  [unwired: 2 in, 1 out]
        n504 = Bundle By Name(cluster=w1133, "Label"="Dorsales" ("Message")) -> (w1132:T1)
        n505 = Insert Into Array(array=cluster{u32, u32}[] [] ("Colors [4]"), new element=w1142) -> (w1135:cluster{u32, u32}[])  [unwired: 1 in]
        n506 = Insert Into Array(array=cluster{u32, u32}[] [] ("Colors [4]"), new element=w1138) -> (w1136:cluster{u32, u32}[])  [unwired: 1 in]
        n507 = Index Array(array=w1125) -> (element=w1131:cluster{u32, u32})  [unwired: 1 in]
        n508 = local write "Master"(FALSE ("Master")) -> ()
        n509 = property on="Gluteos Bool" class="Bool"("Colors [4]"=w1136) -> ()  [unwired: 2 in, 2 out]
        n510 = property on="Abdomen Bool" class="Bool"("Colors [4]"=w1136) -> ()  [unwired: 2 in, 2 out]
        n511 = Unbundle(w1131) -> (w1127:u32)  [unwired: 1 out]
        n512 = property on="Isquiotibiales Bool" class="Bool"("Colors [4]"=w1136) -> ()  [unwired: 2 in, 2 out]
        n513 = property on="Cuadriceps Bool" class="Bool"("Colors [4]"=w1136) -> ()  [unwired: 2 in, 2 out]
        n514 = property on="Dorsales Bool" class="Bool"("Colors [4]"=w1135) -> ()  [unwired: 2 in, 2 out]
        n515 = Bundle(w1127, "Boolean Text.Text Colors:Text Color"=u32 40709) -> (w1130:T2)  [unwired: 1 in]
        n516 = property on="Pectorales Bool" class="Bool"("Colors [4]"=w1136) -> ()  [unwired: 2 in, 2 out]
        n517 = property on="Lumbares Bool" class="Bool"("Colors [4]"=w1136) -> ()  [unwired: 2 in, 2 out]
        n518 = property on="Trapecio Bool" class="Bool"("Colors [4]"=w1136) -> ()  [unwired: 2 in, 2 out]
        n519 = property on="Opcional Bool" class="Bool"("Colors [4]"=w1136) -> ()  [unwired: 2 in, 2 out]
        n520 = property on="Biceps Bool" class="Bool"("Colors [4]"=w1136) -> ()  [unwired: 2 in, 2 out]
        n521 = Replace Array Subset(array=w1125, new element=w1130, index=0) -> (w1124:cluster{u32, u32}[])
        n522 = property on="Master" class="Bool (strict)"(error in=w1122, "Colors [4]"=w1124) -> (error out=w1123:errorcluster)  [unwired: 1 in, 1 out]
        n523 = property on="Master" class="Bool (strict)"(error in=w1123, "BoolText.TextColor"=u32 16448250 ("Boolean Text.Text Colors:Text Color")) -> ()  [unwired: 1 in, 2 out]
      }
      event "Trapecio Bool": Value Change {
        n524 = event-data() -> ()  [unwired: 1 in, 6 out]
        n525 = Bundle By Name(cluster=cluster{"Color Box":u32, "Color Box 2":u32} {"Color Box"=12369084, "Color Box 2"=12369084}, "Color Box"=u32 16711680 ("Color Box 2")) -> (w1167:cluster{"Color Box":u32, "Color Box 2":u32})
        n526 = Bundle By Name(cluster=cluster{"Color Box":u32, "Color Box 2":u32} {"Color Box"=12369084, "Color Box 2"=12369084}, "Color Box"=u32 12369084 ("Color Box 2")) -> (w1163:cluster{"Color Box":u32, "Color Box 2":u32})
        n527 = Bundle By Name(cluster=w1158, "Label"="Trapecio" ("Message")) -> (w1157:T1)
        n528 = property on="Master" class="Bool (strict)"() -> (error out=w1147:errorcluster, "Colors [4]"=w1150:cluster{u32, u32}[])  [unwired: 2 in, 1 out]
        n529 = Insert Into Array(array=cluster{u32, u32}[] [] ("Colors [4]"), new element=w1167) -> (w1160:cluster{u32, u32}[])  [unwired: 1 in]
        n530 = Insert Into Array(array=cluster{u32, u32}[] [] ("Colors [4]"), new element=w1163) -> (w1161:cluster{u32, u32}[])  [unwired: 1 in]
        n531 = local write "Master"(FALSE ("Master")) -> ()
        n532 = property on="Trapecio Bool" class="Bool"("Colors [4]"=w1160) -> ()  [unwired: 2 in, 2 out]
        n533 = property on="Gluteos Bool" class="Bool"("Colors [4]"=w1161) -> ()  [unwired: 2 in, 2 out]
        n534 = property on="Abdomen Bool" class="Bool"("Colors [4]"=w1161) -> ()  [unwired: 2 in, 2 out]
        n535 = Index Array(array=w1150) -> (element=w1156:cluster{u32, u32})  [unwired: 1 in]
        n536 = property on="Isquiotibiales Bool" class="Bool"("Colors [4]"=w1161) -> ()  [unwired: 2 in, 2 out]
        n537 = property on="Cuadriceps Bool" class="Bool"("Colors [4]"=w1161) -> ()  [unwired: 2 in, 2 out]
        n538 = Unbundle(w1156) -> (w1152:u32)  [unwired: 1 out]
        n539 = property on="Pectorales Bool" class="Bool"("Colors [4]"=w1161) -> ()  [unwired: 2 in, 2 out]
        n540 = property on="Lumbares Bool" class="Bool"("Colors [4]"=w1161) -> ()  [unwired: 2 in, 2 out]
        n541 = property on="Dorsales Bool" class="Bool"("Colors [4]"=w1161) -> ()  [unwired: 2 in, 2 out]
        n542 = property on="Opcional Bool" class="Bool"("Colors [4]"=w1161) -> ()  [unwired: 2 in, 2 out]
        n543 = property on="Biceps Bool" class="Bool"("Colors [4]"=w1161) -> ()  [unwired: 2 in, 2 out]
        n544 = Bundle(w1152, "Boolean Text.Text Colors:Text Color"=u32 40709) -> (w1155:T2)  [unwired: 1 in]
        n545 = Replace Array Subset(array=w1150, new element=w1155, index=0) -> (w1149:cluster{u32, u32}[])
        n546 = property on="Master" class="Bool (strict)"(error in=w1147, "Colors [4]"=w1149) -> (error out=w1148:errorcluster)  [unwired: 1 in, 1 out]
        n547 = property on="Master" class="Bool (strict)"(error in=w1148, "BoolText.TextColor"=u32 16448250 ("Boolean Text.Text Colors:Text Color")) -> ()  [unwired: 1 in, 2 out]
      }
      event "Pectorales Bool": Value Change {
        n548 = event-data() -> ()  [unwired: 1 in, 6 out]
        n549 = Bundle By Name(cluster=cluster{"Color Box":u32, "Color Box 2":u32} {"Color Box"=12369084, "Color Box 2"=12369084}, "Color Box"=u32 16711680 ("Color Box 2")) -> (w1192:cluster{"Color Box":u32, "Color Box 2":u32})
        n550 = Bundle By Name(cluster=cluster{"Color Box":u32, "Color Box 2":u32} {"Color Box"=12369084, "Color Box 2"=12369084}, "Color Box"=u32 12369084 ("Color Box 2")) -> (w1188:cluster{"Color Box":u32, "Color Box 2":u32})
        n551 = property on="Master" class="Bool (strict)"() -> (error out=w1172:errorcluster, "Colors [4]"=w1175:cluster{u32, u32}[])  [unwired: 2 in, 1 out]
        n552 = Bundle By Name(cluster=w1183, "Label"="Pectorales" ("Message")) -> (w1182:T1)
        n553 = Insert Into Array(array=cluster{u32, u32}[] [] ("Colors [4]"), new element=w1192) -> (w1185:cluster{u32, u32}[])  [unwired: 1 in]
        n554 = Insert Into Array(array=cluster{u32, u32}[] [] ("Colors [4]"), new element=w1188) -> (w1186:cluster{u32, u32}[])  [unwired: 1 in]
        n555 = local write "Master"(FALSE ("Master")) -> ()
        n556 = Index Array(array=w1175) -> (element=w1181:cluster{u32, u32})  [unwired: 1 in]
        n557 = Unbundle(w1181) -> (w1177:u32)  [unwired: 1 out]
        n558 = property on="Pectorales Bool" class="Bool"("Colors [4]"=w1185) -> ()  [unwired: 2 in, 2 out]
        n559 = property on="Gluteos Bool" class="Bool"("Colors [4]"=w1186) -> ()  [unwired: 2 in, 2 out]
        n560 = property on="Abdomen Bool" class="Bool"("Colors [4]"=w1186) -> ()  [unwired: 2 in, 2 out]
        n561 = property on="Isquiotibiales Bool" class="Bool"("Colors [4]"=w1186) -> ()  [unwired: 2 in, 2 out]
        n562 = property on="Cuadriceps Bool" class="Bool"("Colors [4]"=w1186) -> ()  [unwired: 2 in, 2 out]
        n563 = Bundle(w1177, "Boolean Text.Text Colors:Text Color"=u32 40709) -> (w1180:T2)  [unwired: 1 in]
        n564 = property on="Trapecio Bool" class="Bool"("Colors [4]"=w1186) -> ()  [unwired: 2 in, 2 out]
        n565 = property on="Lumbares Bool" class="Bool"("Colors [4]"=w1186) -> ()  [unwired: 2 in, 2 out]
        n566 = property on="Dorsales Bool" class="Bool"("Colors [4]"=w1186) -> ()  [unwired: 2 in, 2 out]
        n567 = property on="Opcional Bool" class="Bool"("Colors [4]"=w1186) -> ()  [unwired: 2 in, 2 out]
        n568 = property on="Biceps Bool" class="Bool"("Colors [4]"=w1186) -> ()  [unwired: 2 in, 2 out]
        n569 = Replace Array Subset(array=w1175, new element=w1180, index=0) -> (w1174:cluster{u32, u32}[])
        n570 = property on="Master" class="Bool (strict)"(error in=w1172, "Colors [4]"=w1174) -> (error out=w1173:errorcluster)  [unwired: 1 in, 1 out]
        n571 = property on="Master" class="Bool (strict)"(error in=w1173, "BoolText.TextColor"=u32 16448250 ("Boolean Text.Text Colors:Text Color")) -> ()  [unwired: 1 in, 2 out]
      }
      event "Biceps Bool": Value Change {
        n572 = event-data() -> ()  [unwired: 1 in, 6 out]
        n573 = Bundle By Name(cluster=cluster{"Color Box":u32, "Color Box 2":u32} {"Color Box"=12369084, "Color Box 2"=12369084}, "Color Box"=u32 16711680 ("Color Box 2")) -> (w1217:cluster{"Color Box":u32, "Color Box 2":u32})
        n574 = Bundle By Name(cluster=cluster{"Color Box":u32, "Color Box 2":u32} {"Color Box"=12369084, "Color Box 2"=12369084}, "Color Box"=u32 12369084 ("Color Box 2")) -> (w1213:cluster{"Color Box":u32, "Color Box 2":u32})
        n575 = property on="Master" class="Bool (strict)"() -> (error out=w1197:errorcluster, "Colors [4]"=w1200:cluster{u32, u32}[])  [unwired: 2 in, 1 out]
        n576 = Bundle By Name(cluster=w1208, "Label"="Biceps" ("Message")) -> (w1207:T1)
        n577 = Insert Into Array(array=cluster{u32, u32}[] [] ("Colors [4]"), new element=w1217) -> (w1210:cluster{u32, u32}[])  [unwired: 1 in]
        n578 = Insert Into Array(array=cluster{u32, u32}[] [] ("Colors [4]"), new element=w1213) -> (w1211:cluster{u32, u32}[])  [unwired: 1 in]
        n579 = Index Array(array=w1200) -> (element=w1206:cluster{u32, u32})  [unwired: 1 in]
        n580 = local write "Master"(FALSE ("Master")) -> ()
        n581 = Unbundle(w1206) -> (w1202:u32)  [unwired: 1 out]
        n582 = property on="Biceps Bool" class="Bool"("Colors [4]"=w1210) -> ()  [unwired: 2 in, 2 out]
        n583 = property on="Gluteos Bool" class="Bool"("Colors [4]"=w1211) -> ()  [unwired: 2 in, 2 out]
        n584 = property on="Abdomen Bool" class="Bool"("Colors [4]"=w1211) -> ()  [unwired: 2 in, 2 out]
        n585 = property on="Isquiotibiales Bool" class="Bool"("Colors [4]"=w1211) -> ()  [unwired: 2 in, 2 out]
        n586 = property on="Cuadriceps Bool" class="Bool"("Colors [4]"=w1211) -> ()  [unwired: 2 in, 2 out]
        n587 = Bundle(w1202, "Boolean Text.Text Colors:Text Color"=u32 40709) -> (w1205:T2)  [unwired: 1 in]
        n588 = property on="Trapecio Bool" class="Bool"("Colors [4]"=w1211) -> ()  [unwired: 2 in, 2 out]
        n589 = property on="Lumbares Bool" class="Bool"("Colors [4]"=w1211) -> ()  [unwired: 2 in, 2 out]
        n590 = property on="Dorsales Bool" class="Bool"("Colors [4]"=w1211) -> ()  [unwired: 2 in, 2 out]
        n591 = property on="Opcional Bool" class="Bool"("Colors [4]"=w1211) -> ()  [unwired: 2 in, 2 out]
        n592 = property on="Pectorales Bool" class="Bool"("Colors [4]"=w1211) -> ()  [unwired: 2 in, 2 out]
        n593 = Replace Array Subset(array=w1200, new element=w1205, index=0) -> (w1199:cluster{u32, u32}[])
        n594 = property on="Master" class="Bool (strict)"(error in=w1197, "Colors [4]"=w1199) -> (error out=w1198:errorcluster)  [unwired: 1 in, 1 out]
        n595 = property on="Master" class="Bool (strict)"(error in=w1198, "BoolText.TextColor"=u32 16448250 ("Boolean Text.Text Colors:Text Color")) -> ()  [unwired: 1 in, 2 out]
      }
      event "Opcional Bool": Value Change {
        n596 = event-data() -> ()  [unwired: 1 in, 6 out]
        n597 = Bundle By Name(cluster=cluster{"Color Box":u32, "Color Box 2":u32} {"Color Box"=12369084, "Color Box 2"=12369084}, "Color Box"=u32 16711680 ("Color Box 2")) -> (w1242:cluster{"Color Box":u32, "Color Box 2":u32})
        n598 = Bundle By Name(cluster=cluster{"Color Box":u32, "Color Box 2":u32} {"Color Box"=12369084, "Color Box 2"=12369084}, "Color Box"=u32 12369084 ("Color Box 2")) -> (w1238:cluster{"Color Box":u32, "Color Box 2":u32})
        n599 = property on="Master" class="Bool (strict)"() -> (error out=w1222:errorcluster, "Colors [4]"=w1225:cluster{u32, u32}[])  [unwired: 2 in, 1 out]
        n600 = Bundle By Name(cluster=w1233, "Label"="Opcional" ("Message")) -> (w1232:T1)
        n601 = Insert Into Array(array=cluster{u32, u32}[] [] ("Colors [4]"), new element=w1242) -> (w1235:cluster{u32, u32}[])  [unwired: 1 in]
        n602 = Insert Into Array(array=cluster{u32, u32}[] [] ("Colors [4]"), new element=w1238) -> (w1236:cluster{u32, u32}[])  [unwired: 1 in]
        n603 = Index Array(array=w1225) -> (element=w1231:cluster{u32, u32})  [unwired: 1 in]
        n604 = local write "Master"(FALSE ("Master")) -> ()
        n605 = property on="Opcional Bool" class="Bool"("Colors [4]"=w1235) -> ()  [unwired: 2 in, 2 out]
        n606 = Unbundle(w1231) -> (w1227:u32)  [unwired: 1 out]
        n607 = property on="Gluteos Bool" class="Bool"("Colors [4]"=w1236) -> ()  [unwired: 2 in, 2 out]
        n608 = property on="Abdomen Bool" class="Bool"("Colors [4]"=w1236) -> ()  [unwired: 2 in, 2 out]
        n609 = property on="Isquiotibiales Bool" class="Bool"("Colors [4]"=w1236) -> ()  [unwired: 2 in, 2 out]
        n610 = property on="Cuadriceps Bool" class="Bool"("Colors [4]"=w1236) -> ()  [unwired: 2 in, 2 out]
        n611 = Bundle(w1227, "Boolean Text.Text Colors:Text Color"=u32 40709) -> (w1230:T2)  [unwired: 1 in]
        n612 = property on="Trapecio Bool" class="Bool"("Colors [4]"=w1236) -> ()  [unwired: 2 in, 2 out]
        n613 = property on="Lumbares Bool" class="Bool"("Colors [4]"=w1236) -> ()  [unwired: 2 in, 2 out]
        n614 = property on="Dorsales Bool" class="Bool"("Colors [4]"=w1236) -> ()  [unwired: 2 in, 2 out]
        n615 = property on="Biceps Bool" class="Bool"("Colors [4]"=w1236) -> ()  [unwired: 2 in, 2 out]
        n616 = property on="Pectorales Bool" class="Bool"("Colors [4]"=w1236) -> ()  [unwired: 2 in, 2 out]
        n617 = Replace Array Subset(array=w1225, new element=w1230, index=0) -> (w1224:cluster{u32, u32}[])
        n618 = property on="Master" class="Bool (strict)"(error in=w1222, "Colors [4]"=w1224) -> (error out=w1223:errorcluster)  [unwired: 1 in, 1 out]
        n619 = property on="Master" class="Bool (strict)"(error in=w1223, "BoolText.TextColor"=u32 16448250 ("Boolean Text.Text Colors:Text Color")) -> ()  [unwired: 1 in, 2 out]
      }
      event "Add Button": Value Change {
        n620 = event-data() -> ()  [unwired: 1 in, 6 out]
        n621 = Unbundle By Name(w1249) -> ("Label"=w1248:string)
        n622 = case shown="\"Cuadriceps\"" w1248 {
          tunnel: [w1252 w1267 w1280 w1290 w1303 w1316 w1329 w1342 w1355 w1368 w1381 w1394] -> w1250
          tunnel: w1249 -> [w1263 w1276 w1289 w1302 w1315 w1328 w1341 w1354 w1367 w1380 w1393 w1394]
          tunnel: w1247 -> [w1254 w1266 w1279 w1291 w1305 w1318 w1330 w1344 w1357 w1370 w1383 _]
          tunnel: w1246 -> [w1253 w1265 w1278 w1292 w1304 w1317 w1331 w1343 w1356 w1369 w1382 _]
          frame "Cuadriceps" {
            n623 = Unbundle By Name(w1263) -> ("Cuadriceps"=w1255:i32)
            n624 = Greater Or Equal To 0?(x=w1255) -> (x >= 0?=w1260:bool)
            n625 = Less Or Equal?(x=w1255, y=100) -> (x <= y?=w1258:bool)
            n626 = Add(x=w1255, y=5) -> (x+y=w1262:i32)
            n627 = And(x=w1260, y=w1258) -> (x .and. y?=w1259:bool)
            n628 = Select(t=w1262, s=w1259, f=w1255) -> (s? t:f=w1256:i32)
            n629 = Bundle By Name(cluster=w1263, "Cuadriceps"=w1256, "Label"="Cuadriceps") -> (w1252:T1)
            n630 = Enqueue Element At Opposite End(queue=w1253, element=w1252, error in (no error)=w1254) -> ()  [unwired: 1 in, 3 out]
          }
          frame "Isquiotibiales" {
            n631 = Unbundle By Name(w1276) -> ("Isquiotibiales"=w1268:i32)
            n632 = Greater Or Equal To 0?(x=w1268) -> (x >= 0?=w1273:bool)
            n633 = Less Or Equal?(x=w1268, y=100) -> (x <= y?=w1271:bool)
            n634 = Add(x=w1268, y=5) -> (x+y=w1275:i32)
            n635 = And(x=w1273, y=w1271) -> (x .and. y?=w1272:bool)
            n636 = Select(t=w1275, s=w1272, f=w1268) -> (s? t:f=w1269:i32)
            n637 = Bundle By Name(cluster=w1276, "Isquiotibiales"=w1269, "Label"="Isquiotibiales") -> (w1267:T1)
            n638 = Enqueue Element At Opposite End(queue=w1265, element=w1267, error in (no error)=w1266) -> ()  [unwired: 1 in, 3 out]
          }
          frame "Gluteos" {
            n639 = Unbundle By Name(w1289) -> ("Gluteos"=w1281:i32)
            n640 = Greater Or Equal To 0?(x=w1281) -> (x >= 0?=w1286:bool)
            n641 = Less Or Equal?(x=w1281, y=100) -> (x <= y?=w1284:bool)
            n642 = Add(x=w1281, y=5) -> (x+y=w1288:i32)
            n643 = And(x=w1286, y=w1284) -> (x .and. y?=w1285:bool)
            n644 = Select(t=w1288, s=w1285, f=w1281) -> (s? t:f=w1282:i32)
            n645 = Bundle By Name(cluster=w1289, "Gluteos"=w1282, "Label"="Gluteos") -> (w1280:T1)
            n646 = Enqueue Element At Opposite End(queue=w1278, element=w1280, error in (no error)=w1279) -> ()  [unwired: 1 in, 3 out]
          }
          frame "Abdomen" {
            n647 = Unbundle By Name(w1302) -> ("Abdomen"=w1294:i32)
            n648 = Greater Or Equal To 0?(x=w1294) -> (x >= 0?=w1299:bool)
            n649 = Less Or Equal?(x=w1294, y=100) -> (x <= y?=w1297:bool)
            n650 = Add(x=w1294, y=5) -> (x+y=w1301:i32)
            n651 = And(x=w1299, y=w1297) -> (x .and. y?=w1298:bool)
            n652 = Select(t=w1301, s=w1298, f=w1294) -> (s? t:f=w1295:i32)
            n653 = Bundle By Name(cluster=w1302, "Abdomen"=w1295, "Label"="Abdomen") -> (w1290:T1)
            n654 = Enqueue Element At Opposite End(queue=w1292, element=w1290, error in (no error)=w1291) -> ()  [unwired: 1 in, 3 out]
          }
          frame "Lumbares" {
            n655 = Unbundle By Name(w1315) -> ("Lumbares"=w1307:i32)
            n656 = Greater Or Equal To 0?(x=w1307) -> (x >= 0?=w1312:bool)
            n657 = Less Or Equal?(x=w1307, y=100) -> (x <= y?=w1310:bool)
            n658 = Add(x=w1307, y=5) -> (x+y=w1314:i32)
            n659 = And(x=w1312, y=w1310) -> (x .and. y?=w1311:bool)
            n660 = Select(t=w1314, s=w1311, f=w1307) -> (s? t:f=w1308:i32)
            n661 = Bundle By Name(cluster=w1315, "Lumbares"=w1308, "Label"="Lumbares") -> (w1303:T1)
            n662 = Enqueue Element At Opposite End(queue=w1304, element=w1303, error in (no error)=w1305) -> ()  [unwired: 1 in, 3 out]
          }
          frame "Dorsales" {
            n663 = Unbundle By Name(w1328) -> ("Dorsales"=w1320:i32)
            n664 = Greater Or Equal To 0?(x=w1320) -> (x >= 0?=w1325:bool)
            n665 = Less Or Equal?(x=w1320, y=100) -> (x <= y?=w1323:bool)
            n666 = Add(x=w1320, y=5) -> (x+y=w1327:i32)
            n667 = And(x=w1325, y=w1323) -> (x .and. y?=w1324:bool)
            n668 = Select(t=w1327, s=w1324, f=w1320) -> (s? t:f=w1321:i32)
            n669 = Bundle By Name(cluster=w1328, "Dorsales"=w1321, "Label"="Dorsales") -> (w1316:T1)
            n670 = Enqueue Element At Opposite End(queue=w1317, element=w1316, error in (no error)=w1318) -> ()  [unwired: 1 in, 3 out]
          }
          frame "Trapecio" {
            n671 = Unbundle By Name(w1341) -> ("Trapecio"=w1333:i32)
            n672 = Greater Or Equal To 0?(x=w1333) -> (x >= 0?=w1338:bool)
            n673 = Less Or Equal?(x=w1333, y=100) -> (x <= y?=w1336:bool)
            n674 = Add(x=w1333, y=5) -> (x+y=w1340:i32)
            n675 = And(x=w1338, y=w1336) -> (x .and. y?=w1337:bool)
            n676 = Select(t=w1340, s=w1337, f=w1333) -> (s? t:f=w1334:i32)
            n677 = Bundle By Name(cluster=w1341, "Trapecio"=w1334, "Label"="Trapecio") -> (w1329:T1)
            n678 = Enqueue Element At Opposite End(queue=w1331, element=w1329, error in (no error)=w1330) -> ()  [unwired: 1 in, 3 out]
          }
          frame "Pectorales" {
            n679 = Unbundle By Name(w1354) -> ("Pectorales"=w1346:i32)
            n680 = Greater Or Equal To 0?(x=w1346) -> (x >= 0?=w1351:bool)
            n681 = Less Or Equal?(x=w1346, y=100) -> (x <= y?=w1349:bool)
            n682 = Add(x=w1346, y=5) -> (x+y=w1353:i32)
            n683 = And(x=w1351, y=w1349) -> (x .and. y?=w1350:bool)
            n684 = Select(t=w1353, s=w1350, f=w1346) -> (s? t:f=w1347:i32)
            n685 = Bundle By Name(cluster=w1354, "Pectorales"=w1347, "Label"="Pectorales") -> (w1342:T1)
            n686 = Enqueue Element At Opposite End(queue=w1343, element=w1342, error in (no error)=w1344) -> ()  [unwired: 1 in, 3 out]
          }
          frame "Biceps" {
            n687 = Unbundle By Name(w1367) -> ("Biceps"=w1359:i32)
            n688 = Greater Or Equal To 0?(x=w1359) -> (x >= 0?=w1364:bool)
            n689 = Less Or Equal?(x=w1359, y=100) -> (x <= y?=w1362:bool)
            n690 = Add(x=w1359, y=5) -> (x+y=w1366:i32)
            n691 = And(x=w1364, y=w1362) -> (x .and. y?=w1363:bool)
            n692 = Select(t=w1366, s=w1363, f=w1359) -> (s? t:f=w1360:i32)
            n693 = Bundle By Name(cluster=w1367, "Biceps"=w1360, "Label"="Biceps") -> (w1355:T1)
            n694 = Enqueue Element At Opposite End(queue=w1356, element=w1355, error in (no error)=w1357) -> ()  [unwired: 1 in, 3 out]
          }
          frame "Opcional" {
            n695 = Unbundle By Name(w1380) -> ("Opcional"=w1372:i32)
            n696 = Greater Or Equal To 0?(x=w1372) -> (x >= 0?=w1377:bool)
            n697 = Less Or Equal?(x=w1372, y=100) -> (x <= y?=w1375:bool)
            n698 = Add(x=w1372, y=5) -> (x+y=w1379:i32)
            n699 = And(x=w1377, y=w1375) -> (x .and. y?=w1376:bool)
            n700 = Select(t=w1379, s=w1376, f=w1372) -> (s? t:f=w1373:i32)
            n701 = Bundle By Name(cluster=w1380, "Opcional"=w1373, "Label"="Opcional") -> (w1368:T1)
            n702 = Enqueue Element At Opposite End(queue=w1369, element=w1368, error in (no error)=w1370) -> ()  [unwired: 1 in, 3 out]
          }
          frame "Master" {
            n703 = Unbundle By Name(w1393) -> ("Master"=w1385:i32)
            n704 = Greater Or Equal To 0?(x=w1385) -> (x >= 0?=w1390:bool)
            n705 = Less?(x=w1385, y=100) -> (x < y?=w1388:bool)
            n706 = Add(x=w1385, y=5) -> (x+y=w1392:i32)
            n707 = And(x=w1390, y=w1388) -> (x .and. y?=w1389:bool)
            n708 = Select(t=w1392, s=w1389, f=w1385) -> (s? t:f=w1386:i32)
            n709 = Bundle By Name(cluster=w1393, "Master"=w1386, "Label"="Master") -> (w1381:T1)
            n710 = Enqueue Element At Opposite End(queue=w1382, element=w1381, error in (no error)=w1383) -> ()  [unwired: 1 in, 3 out]
          }
          frame Default {
          }
        }
      }
      event "Remove Button": Value Change {
        n711 = event-data() -> ()  [unwired: 1 in, 6 out]
        n712 = Unbundle By Name(w1398) -> ("Label"=w1397:string)
        n713 = case shown="\"Cuadriceps\"" w1397 {
          tunnel: [w1400 w1411 w1420 w1430 w1440 w1450 w1461 w1470 w1480 w1490 w1500 w1510] -> w1399
          tunnel: w1398 -> [w1409 w1419 w1429 w1439 w1449 w1459 w1469 w1479 w1489 w1499 w1509 w1510]
          tunnel: w1396 -> [w1401 w1412 w1421 w1431 w1442 w1451 w1463 w1471 w1482 w1492 w1502 _]
          tunnel: w1395 -> [w1402 w1413 w1422 w1432 w1441 w1452 w1462 w1472 w1481 w1491 w1501 _]
          frame "Cuadriceps" {
            n714 = Unbundle By Name(w1409) -> ("Cuadriceps"=w1404:i32)
            n715 = Greater Than 0?(x=w1404) -> (x > 0?=w1406:bool)
            n716 = Subtract(x=w1404, y=5) -> (x-y=w1407:i32)
            n717 = Select(t=w1407, s=w1406, f=w1404) -> (s? t:f=w1405:i32)
            n718 = Bundle By Name(cluster=w1409, "Cuadriceps"=w1405, "Label"="Cuadriceps") -> (w1400:T1)
            n719 = Enqueue Element At Opposite End(queue=w1401, element=w1400, error in (no error)=w1402) -> ()  [unwired: 1 in, 3 out]
          }
          frame "Isquiotibiales" {
            n720 = Unbundle By Name(w1419) -> ("Isquiotibiales"=w1414:i32)
            n721 = Greater Than 0?(x=w1414) -> (x > 0?=w1416:bool)
            n722 = Subtract(x=w1414, y=5) -> (x-y=w1417:i32)
            n723 = Select(t=w1417, s=w1416, f=w1414) -> (s? t:f=w1415:i32)
            n724 = Bundle By Name(cluster=w1419, "Isquiotibiales"=w1415, "Label"="Isquiotibiales") -> (w1411:T1)
            n725 = Enqueue Element At Opposite End(queue=w1412, element=w1411, error in (no error)=w1413) -> ()  [unwired: 1 in, 3 out]
          }
          frame "Gluteos" {
            n726 = Unbundle By Name(w1429) -> ("Gluteos"=w1424:i32)
            n727 = Greater Than 0?(x=w1424) -> (x > 0?=w1426:bool)
            n728 = Subtract(x=w1424, y=5) -> (x-y=w1427:i32)
            n729 = Select(t=w1427, s=w1426, f=w1424) -> (s? t:f=w1425:i32)
            n730 = Bundle By Name(cluster=w1429, "Gluteos"=w1425, "Label"="Gluteos") -> (w1420:T1)
            n731 = Enqueue Element At Opposite End(queue=w1421, element=w1420, error in (no error)=w1422) -> ()  [unwired: 1 in, 3 out]
          }
          frame "Abdomen" {
            n732 = Unbundle By Name(w1439) -> ("Abdomen"=w1434:i32)
            n733 = Greater Than 0?(x=w1434) -> (x > 0?=w1436:bool)
            n734 = Subtract(x=w1434, y=5) -> (x-y=w1437:i32)
            n735 = Select(t=w1437, s=w1436, f=w1434) -> (s? t:f=w1435:i32)
            n736 = Bundle By Name(cluster=w1439, "Abdomen"=w1435, "Label"="Abdomen") -> (w1430:T1)
            n737 = Enqueue Element At Opposite End(queue=w1431, element=w1430, error in (no error)=w1432) -> ()  [unwired: 1 in, 3 out]
          }
          frame "Lumbares" {
            n738 = Unbundle By Name(w1449) -> ("Lumbares"=w1444:i32)
            n739 = Greater Than 0?(x=w1444) -> (x > 0?=w1446:bool)
            n740 = Subtract(x=w1444, y=5) -> (x-y=w1447:i32)
            n741 = Select(t=w1447, s=w1446, f=w1444) -> (s? t:f=w1445:i32)
            n742 = Bundle By Name(cluster=w1449, "Lumbares"=w1445, "Label"="Lumbares") -> (w1440:T1)
            n743 = Enqueue Element At Opposite End(queue=w1442, element=w1440, error in (no error)=w1441) -> ()  [unwired: 1 in, 3 out]
          }
          frame "Dorsales" {
            n744 = Unbundle By Name(w1459) -> ("Dorsales"=w1454:i32)
            n745 = Greater Than 0?(x=w1454) -> (x > 0?=w1456:bool)
            n746 = Subtract(x=w1454, y=5) -> (x-y=w1457:i32)
            n747 = Select(t=w1457, s=w1456, f=w1454) -> (s? t:f=w1455:i32)
            n748 = Bundle By Name(cluster=w1459, "Dorsales"=w1455, "Label"="Dorsales") -> (w1450:T1)
            n749 = Enqueue Element At Opposite End(queue=w1451, element=w1450, error in (no error)=w1452) -> ()  [unwired: 1 in, 3 out]
          }
          frame "Trapecio" {
            n750 = Unbundle By Name(w1469) -> ("Trapecio"=w1464:i32)
            n751 = Greater Than 0?(x=w1464) -> (x > 0?=w1466:bool)
            n752 = Subtract(x=w1464, y=5) -> (x-y=w1467:i32)
            n753 = Select(t=w1467, s=w1466, f=w1464) -> (s? t:f=w1465:i32)
            n754 = Bundle By Name(cluster=w1469, "Trapecio"=w1465, "Label"="Trapecio") -> (w1461:T1)
            n755 = Enqueue Element At Opposite End(queue=w1463, element=w1461, error in (no error)=w1462) -> ()  [unwired: 1 in, 3 out]
          }
          frame "Pectorales" {
            n756 = Unbundle By Name(w1479) -> ("Pectorales"=w1474:i32)
            n757 = Greater Than 0?(x=w1474) -> (x > 0?=w1476:bool)
            n758 = Subtract(x=w1474, y=5) -> (x-y=w1477:i32)
            n759 = Select(t=w1477, s=w1476, f=w1474) -> (s? t:f=w1475:i32)
            n760 = Bundle By Name(cluster=w1479, "Pectorales"=w1475, "Label"="Pectorales") -> (w1470:T1)
            n761 = Enqueue Element At Opposite End(queue=w1471, element=w1470, error in (no error)=w1472) -> ()  [unwired: 1 in, 3 out]
          }
          frame "Biceps" {
            n762 = Unbundle By Name(w1489) -> ("Biceps"=w1484:i32)
            n763 = Greater Than 0?(x=w1484) -> (x > 0?=w1486:bool)
            n764 = Subtract(x=w1484, y=5) -> (x-y=w1487:i32)
            n765 = Select(t=w1487, s=w1486, f=w1484) -> (s? t:f=w1485:i32)
            n766 = Bundle By Name(cluster=w1489, "Biceps"=w1485, "Label"="Biceps") -> (w1480:T1)
            n767 = Enqueue Element At Opposite End(queue=w1482, element=w1480, error in (no error)=w1481) -> ()  [unwired: 1 in, 3 out]
          }
          frame "Opcional" {
            n768 = Unbundle By Name(w1499) -> ("Opcional"=w1494:i32)
            n769 = Greater Than 0?(x=w1494) -> (x > 0?=w1496:bool)
            n770 = Subtract(x=w1494, y=5) -> (x-y=w1497:i32)
            n771 = Select(t=w1497, s=w1496, f=w1494) -> (s? t:f=w1495:i32)
            n772 = Bundle By Name(cluster=w1499, "Opcional"=w1495, "Label"="Opcional") -> (w1490:T1)
            n773 = Enqueue Element At Opposite End(queue=w1492, element=w1490, error in (no error)=w1491) -> ()  [unwired: 1 in, 3 out]
          }
          frame "Master" {
            n774 = Unbundle By Name(w1509) -> ("Master"=w1504:i32)
            n775 = Greater Than 0?(x=w1504) -> (x > 0?=w1506:bool)
            n776 = Subtract(x=w1504, y=5) -> (x-y=w1507:i32)
            n777 = Select(t=w1507, s=w1506, f=w1504) -> (s? t:f=w1505:i32)
            n778 = Bundle By Name(cluster=w1509, "Master"=w1505, "Label"="Master") -> (w1500:T1)
            n779 = Enqueue Element At Opposite End(queue=w1502, element=w1500, error in (no error)=w1501) -> ()  [unwired: 1 in, 3 out]
          }
          frame Default {
          }
        }
      }
      event "Slider": Value Change {
        n780 = event-data() -> ()  [unwired: 1 in, 6 out]
        n781 = Unbundle By Name(w1515) -> ("Label"=w1513:string)
        n782 = case shown="\"Cuadriceps\"" w1513 {
          tunnel: [w1517 w1523 w1529 w1535 w1541 w1547 w1553 w1559 w1565 w1571 w1577 w1584] -> w1516
          tunnel: w1515 -> [w1522 w1528 w1534 w1540 w1546 w1552 w1558 w1564 w1570 w1576 w1582 w1585]
          tunnel: "Slider" -> [w1521 w1527 w1533 w1539 w1545 w1551 w1557 w1563 w1569 w1575 w1581 w1583]
          tunnel: w1512 -> [w1518 w1525 w1531 w1537 w1542 w1549 w1555 w1561 w1567 w1573 w1579 _]
          tunnel: w1511 -> [w1519 w1524 w1530 w1536 w1543 w1548 w1554 w1560 w1566 w1572 w1578 _]
          frame "Cuadriceps" {
            n783 = Bundle By Name(cluster=w1522, "Cuadriceps"=w1521, "Label"="Cuadriceps") -> (w1517:T1)
            n784 = Enqueue Element At Opposite End(queue=w1519, element=w1517, error in (no error)=w1518) -> ()  [unwired: 1 in, 3 out]
          }
          frame "Isquiotibiales" {
            n785 = Bundle By Name(cluster=w1528, "Isquiotibiales"=w1527, "Label"="Isquiotibiales") -> (w1523:T1)
            n786 = Enqueue Element At Opposite End(queue=w1524, element=w1523, error in (no error)=w1525) -> ()  [unwired: 1 in, 3 out]
          }
          frame "Gluteos" {
            n787 = Bundle By Name(cluster=w1534, "Gluteos"=w1533, "Label"="Gluteos") -> (w1529:T1)
            n788 = Enqueue Element At Opposite End(queue=w1530, element=w1529, error in (no error)=w1531) -> ()  [unwired: 1 in, 3 out]
          }
          frame "Abdomen" {
            n789 = Bundle By Name(cluster=w1540, "Abdomen"=w1539, "Label"="Abdomen") -> (w1535:T1)
            n790 = Enqueue Element At Opposite End(queue=w1536, element=w1535, error in (no error)=w1537) -> ()  [unwired: 1 in, 3 out]
          }
          frame "Lumbares" {
            n791 = Bundle By Name(cluster=w1546, "Lumbares"=w1545, "Label"="Lumbares") -> (w1541:T1)
            n792 = Enqueue Element At Opposite End(queue=w1543, element=w1541, error in (no error)=w1542) -> ()  [unwired: 1 in, 3 out]
          }
          frame "Dorsales" {
            n793 = Bundle By Name(cluster=w1552, "Dorsales"=w1551, "Label"="Dorsales") -> (w1547:T1)
            n794 = Enqueue Element At Opposite End(queue=w1548, element=w1547, error in (no error)=w1549) -> ()  [unwired: 1 in, 3 out]
          }
          frame "Trapecio" {
            n795 = Bundle By Name(cluster=w1558, "Trapecio"=w1557, "Label"="Trapecio") -> (w1553:T1)
            n796 = Enqueue Element At Opposite End(queue=w1554, element=w1553, error in (no error)=w1555) -> ()  [unwired: 1 in, 3 out]
          }
          frame "Pectorales" {
            n797 = Bundle By Name(cluster=w1564, "Pectorales"=w1563, "Label"="Pectorales") -> (w1559:T1)
            n798 = Enqueue Element At Opposite End(queue=w1560, element=w1559, error in (no error)=w1561) -> ()  [unwired: 1 in, 3 out]
          }
          frame "Biceps" {
            n799 = Bundle By Name(cluster=w1570, "Biceps"=w1569, "Label"="Biceps") -> (w1565:T1)
            n800 = Enqueue Element At Opposite End(queue=w1566, element=w1565, error in (no error)=w1567) -> ()  [unwired: 1 in, 3 out]
          }
          frame "Opcional" {
            n801 = Bundle By Name(cluster=w1576, "Opcional"=w1575, "Label"="Opcional") -> (w1571:T1)
            n802 = Enqueue Element At Opposite End(queue=w1572, element=w1571, error in (no error)=w1573) -> ()  [unwired: 1 in, 3 out]
          }
          frame "Master" {
            n803 = Bundle By Name(cluster=w1582, "Master"=w1581, "Label"="Master") -> (w1577:T1)
            n804 = Enqueue Element At Opposite End(queue=w1578, element=w1577, error in (no error)=w1579) -> ()  [unwired: 1 in, 3 out]
          }
          frame "Inicio", Default {
            n805 = Bundle By Name(cluster=w1585, "Slider"=w1583) -> (w1584:T1)
          }
        }
      }
      event "Back": Value Change {
        n806 = event-data() -> ()  [unwired: 1 in, 6 out]
        n807 = Bundle By Name(cluster=w1588, "Label"="Back" ("Message")) -> (w1586:T1)
      }
      event "Master": Value Change {
        n808 = event-data() -> ()  [unwired: 1 in, 6 out]
        n809 = property on="Master" class="Bool (strict)"() -> ("Colors [4]"=w1596:cluster{u32, u32}[])  [unwired: 2 in, 2 out]
        n810 = Index Array(array=w1596) -> (element=w1597:cluster{u32, u32})  [unwired: 1 in]
        n811 = Unbundle(w1597) -> (w1594:u32, w1593:u32)
        n812 = case shown="True" "Master" {
          tunnel: [u32 16448250 ("Boolean Text.Text Colors:Text Color") u32 0 ("Boolean Text.Text Colors:Text Color")] -> w1598
          tunnel: w1594 -> [w1604 w1613]
          tunnel: w1593 -> [_ _]
          tunnel: w1596 -> [w1608 w1615]
          tunnel: [w1605 w1616] -> w1595
          tunnel: w1591 -> [w1602 w1611]
          tunnel: [w1601 w1610] -> w1590
          frame False {
            n813 = Bundle(w1604, "Boolean Text.Text Colors:Text Color"=u32 40709) -> (w1607:T2)  [unwired: 1 in]
            n814 = Bundle By Name(cluster=w1602, "Label"="Inicio") -> (w1601:T1)
            n815 = Replace Array Subset(array=w1608, new element=w1607, index=0) -> (w1605:cluster{u32, u32}[])
          }
          frame True {
            n816 = Bundle(w1613, "Boolean Text.Text Colors:Text Color"=u32 16711680) -> (w1618:T2)  [unwired: 1 in]
            n817 = Bundle By Name(cluster=w1611, "Label"="Master" ("Message")) -> (w1610:T1)
            n818 = Replace Array Subset(array=w1615, new element=w1618, index=0) -> (w1616:cluster{u32, u32}[])
          }
        }
        n819 = property on="Master" class="Bool (strict)"("BoolText.TextColor"=w1598) -> ()  [unwired: 2 in, 2 out]
        n820 = property on="Master" class="Bool (strict)"("Colors [4]"=w1595) -> ()  [unwired: 2 in, 2 out]
        "Master?" <- "Master"
      }
      event "Help": Value Change {
        n821 = event-data() -> ()  [unwired: 1 in, 6 out]
        n822 = call "Help.vi"() -> ()  [unwired: 11 in, 1 out]
      }
      event "Impulso": Value Change {
        n823 = event-data() -> ()  [unwired: 1 in, 6 out]
        n824 = Unbundle By Name(w1629) -> ("Tiempo"=w1627:i32, "Impulso"=w1628:i32, "Ruptura"=w1626:i32, "Frecuencia"=w1625:i32, "Profundidad"=w1624:i32, "Ganancia"=w1623:dbl)
        n825 = Build Array(w1627, w1628, w1626, w1625, w1624, w1623) -> (w1622:dbl[])
        n826 = call "Impulso.vi"("appended array"=w1622) -> ("Parametros"=w1650:cluster{i32, i32, i32, i32, i32, dbl})  [unwired: 1 in]
        n827 = Unbundle(w1650) -> (w1633:i32, w1631:i32, w1632:i32, w1643:i32, w1637:i32, w1640:dbl)
        n828 = Bundle By Name(cluster=w1629, "Label"="Frecuencia" ("Message"), "Frecuencia"=w1643) -> (w1642:T1)
        n829 = Enqueue Element(queue=w1649, element=w1642, error in (no error)=w1648) -> (queue out=w1646:refnum<queue>, error out=w1647:errorcluster)  [unwired: 1 in, 1 out]
        n830 = Bundle By Name(cluster=w1642, "Label"="Ganancia", "Ganancia"=w1640) -> (w1639:T1)
        n831 = Enqueue Element(queue=w1646, element=w1639, error in (no error)=w1647) -> (queue out=w1644:refnum<queue>, error out=w1645:errorcluster)  [unwired: 1 in, 1 out]
        n832 = Bundle By Name(cluster=w1639, "Label"="Impulso", "Profundidad"=w1637) -> (w1635:T1)
        n833 = Enqueue Element(queue=w1644, element=w1635, error in (no error)=w1645) -> (error out=w1636:errorcluster)  [unwired: 1 in, 2 out]
        n834 = Bundle By Name(cluster=w1635, "Label"="Inicio", "Tiempo"=w1633, "Ruptura"=w1632, "Impulso"=w1631) -> (w1634:T1)
      }
      event "Reset": Value Change {
        n835 = event-data() -> ()  [unwired: 1 in, 6 out]
        n836 = Bundle By Name(cluster=w1702, "Label"="Cuadriceps" ("Message"), "Cuadriceps"=0) -> (w1695:T1)
        n837 = Enqueue Element At Opposite End(queue=w1701, element=w1695, error in (no error)=w1700) -> (queue out=w1698:refnum<queue>, error out=w1699:errorcluster)  [unwired: 1 in, 1 out]
        n838 = Bundle By Name(cluster=w1695, "Label"="Isquiotibiales", "Isquiotibiales"=0) -> (w1693:T1)
        n839 = Enqueue Element At Opposite End(queue=w1698, element=w1693, error in (no error)=w1699) -> (queue out=w1696:refnum<queue>, error out=w1697:errorcluster)  [unwired: 1 in, 1 out]
        n840 = Bundle By Name(cluster=w1693, "Label"="Gluteos", "Gluteos"=0) -> (w1684:T1)
        n841 = Enqueue Element At Opposite End(queue=w1696, element=w1684, error in (no error)=w1697) -> (queue out=w1687:refnum<queue>, error out=w1688:errorcluster)  [unwired: 1 in, 1 out]
        n842 = Bundle By Name(cluster=w1684, "Label"="Abdomen", "Abdomen"=0) -> (w1681:T1)
        n843 = Enqueue Element At Opposite End(queue=w1687, element=w1681, error in (no error)=w1688) -> (queue out=w1685:refnum<queue>, error out=w1686:errorcluster)  [unwired: 1 in, 1 out]
        n844 = Bundle By Name(cluster=w1681, "Label"="Lumbares", "Lumbares"=0) -> (w1678:T1)
        n845 = Enqueue Element At Opposite End(queue=w1685, element=w1678, error in (no error)=w1686) -> (queue out=w1674:refnum<queue>, error out=w1675:errorcluster)  [unwired: 1 in, 1 out]
        n846 = Bundle By Name(cluster=w1678, "Label"="Dorsales", "Dorsales"=0) -> (w1671:T1)
        n847 = Bundle By Name(cluster=w1671, "Label"="Trapecio", "Trapecio"=0) -> (w1668:T1)
        n848 = Enqueue Element At Opposite End(queue=w1674, element=w1671, error in (no error)=w1675) -> (queue out=w1672:refnum<queue>, error out=w1673:errorcluster)  [unwired: 1 in, 1 out]
        n849 = Enqueue Element At Opposite End(queue=w1672, element=w1668, error in (no error)=w1673) -> (queue out=w1665:refnum<queue>, error out=w1664:errorcluster)  [unwired: 1 in, 1 out]
        n850 = Bundle By Name(cluster=w1668, "Label"="Pectorales", "Pectorales"=0) -> (w1663:T1)
        n851 = Bundle By Name(cluster=w1663, "Label"="Biceps", "Biceps"=0) -> (w1658:T1)
        n852 = Enqueue Element At Opposite End(queue=w1665, element=w1663, error in (no error)=w1664) -> (queue out=w1659:refnum<queue>, error out=w1660:errorcluster)  [unwired: 1 in, 1 out]
        n853 = Enqueue Element At Opposite End(queue=w1659, element=w1658, error in (no error)=w1660) -> (queue out=w1654:refnum<queue>, error out=w1655:errorcluster)  [unwired: 1 in, 1 out]
        n854 = Bundle By Name(cluster=w1658, "Label"="Opcional", "Opcional"=0) -> (w1653:T1)
        n855 = Enqueue Element At Opposite End(queue=w1654, element=w1653, error in (no error)=w1655) -> ()  [unwired: 1 in, 3 out]
      }
      event "Start": Value Change {
        n856 = event-data() -> ()  [unwired: 1 in, 6 out]
        n857 = Bundle By Name(cluster=w1711, "Label"="Start" ("Message")) -> (w1710:T1)
        n858 = case shown="True" "Start" {
          tunnel: w1707 -> [w1715 _]
          tunnel: w1706 -> [w1714 w1716]
          tunnel: [w1713 w1716] -> w1705
          frame False {
            n859 = Flush Queue(queue=w1715, error in (no error)=w1714) -> (error out=w1713:errorcluster)  [unwired: 2 out]
          }
          frame True {
          }
        }
        "Start?" <- "Start"
      }
    }
    "Cluster" <- w868
  }
  n860 = Release Queue(queue=w8, error in (no error)=w2) -> ()  [unwired: 1 in, 3 out]
  n861 = VISA Close(VISA resource name=w5, error in (no error)=w4) -> (error out=→"error out 2":errorcluster)
  "error out" <- "error in (no error)"
